vi "Controle_Manip_Main_GUI_Backup1.vi"() -> ()   [LabVIEW 2019]
doc: "VI for micro-photoluminescence setup in GH013 to study the emission properties of single nanoemitters in the visible range."
uses:
  subVIs/TypeDefs/AcqMode.ctl
  D:/Users/manip-thz/Documents/Controle_Manip_2020/Thorlabs.MotionControl.Controls.dll
  Thorlabs.MotionControl.Controls.dll
  D:/Users/manip-thz/Documents/Controle_Manip_2020/Thorlabs.MotionControl.KCube.SolenoidCLI.dll
  Thorlabs.MotionControl.KCube.SolenoidCLI.dll
  D:/Users/manip-thz/Documents/Controle_Manip_2020/Thorlabs.MotionControl.KCube.PiezoCLI.dll
  Thorlabs.MotionControl.KCube.PiezoCLI.dll
  subVIs/Light Field/lightfield-automation-labview/LightField Automation.lvclass
  subVIs/Light Field/lightfield-automation-labview/VIs/TypeDefs/OpticalPortLocation.ctl
  System.Windows.Forms
  C:/Program Files/Thorlabs/Scientific Imaging/DCx Camera Support/Develop/DotNet/uc480DotNet.dll
  <vilib>/DAQmx/write.llb/DAQmx Write (Analog DBL 1Chan 1Samp).vi
  <vilib>/DAQmx/create/channels.llb/DAQmx Create Channel (AO-Voltage-Basic).vi
  <vilib>/DAQmx/miscellaneous.llb/DAQmx Fill In Error Info.vi
  subVIs/Newport/Newport ESP301/Newport ESP301.lvlib
panel:
  out "Thorcam Error":errorcluster caption="Error Out"
  out "ThorCam Reference":refnum<k24>
  out "Shutter Ctrls":u16(ring)
  out "Serial Number":string
  out "Scan XY Map Params":refnum<vi>[](array[refnum])
  in  "Diode Driver Error":errorcluster caption="error in (no error)" {"code" format="%.0x"}
  out "Color":u32(colorbox)=4980812
  out "Laser on?":bool
  out "Angles":dbl[](array[numeric])
  out "Scan Polar Params":refnum<vi>[](array[refnum])
  in  "ESP 301 Error":errorcluster
  in  "ESP300 Error":errorcluster
  out "Data":T1(array[cluster])
  out "Wavelength calibration":dbl[](array[numeric])
  out "LightField Automation error out":errorcluster
  out "LightField Automation out":refnum<class "LightField Automation.lvclass">
  out "Photodiode error out":errorcluster caption="error out" {"code" format="%.0x"}
  out "Photodiode handle out":refnum<visa-resource-name> caption="instrument handle out"
  out "KCubePiezoControl X Reference":refnum<k24>
  out "KCubePiezoDevice X Reference":refnum<k24>
  out "KCubePiezoDevice Y Reference":refnum<k24>
  out "KCubePiezoControl Y Reference":refnum<k24>
  out "KCubePiezoControl Z Reference":refnum<k24>
  out "KCubePiezoDevice Z Reference":refnum<k24>
  out "KCube Shutter Device Reference":refnum<k24>
  in  "Shutter mode":bool
  out "KCubeSolenoidControl Reference":refnum<k24>
  in  "Cryostat":enum16{"Montana", "Oxford"}(ring) caption="Cryo :"
  out "Excitation Power (uW)":dbl=0.2 caption="P    =" format="%#_3p"
  in  "Acq Time (ms)":dbl=500.0 caption="Acq Time :" min=0.0 max=360000.0 step=50.0
  in  "Auto< ?":bool
  in  "Acq Mode":T2=enum."Spectrum" caption="Acquire :"
  in  "Comment":string
  out "Log file":string caption="Status"
  in  "Experiment Name":string="B1802CF_QD0"
  in  "Experiment Graph Controls":T3(tab)
  in  "CCD 1D Spectrum Main  Cursor2WL 2 Mono 2":bool caption="CCD 1D Spectrum Main  Cursor2WL"
  in  "CCD 1D Spectrum Main  Cursor2WL 1 Mono 2":bool caption="CCD 1D Spectrum Main  Cursor2WL"
  in  "CCD 1D Spectrum Main  Cursor2WL 2 Mono 1":bool caption="CCD 1D Spectrum Main  Cursor2WL"
  in  "CCD 1D Spectrum Main  Cursor2WL 1 Mono 1":bool caption="CCD 1D Spectrum Main  Cursor2WL"
  out "CCD 1D Spectrum Main Cursor 1 nm":dbl caption="nm"
  out "CCD 1D Spectrum Main Cursor 2 nm":dbl caption="nm"
  in  "Full scale":bool
  in  "Acquire Continuous Spectrum":bool
  in  "Acquire Spectrum":bool
  out "CCD 2D Image Main":dbl[][](graph)
  in  "Save Spectrum N":bool
  in  "Save Spectrum":bool
  out "CCD 1D Spectrum Main":cluster{dbl[], dbl[]}(graph)
  in  "Stop continuous":bool
  out "CCD 1D Spectrum Main Energy Scale":cluster{dbl[], dbl[]}(graph)
  out "CCD 1D Spectrum Main Cursor":dbl caption="eV" format="%#_6p"
  out "CCD 1D Spectrum Main Cursor 2":dbl caption="eV" format="%#_6p"
  out "CCD 1D Spectrum Main deltaE":dbl caption="eV" format="%#_3p"
  out "CCD 1D Spectrum Main deltanm":dbl caption="m" format="%#_3p"
  out "XY Intensity Map":dbl[][](graph)=[[3.904687043201515e-13, 6.684989195773002e-11, 3.649880430807626e-09, 6.355065252727497e-08, 3.5287820878809013e-07, 6.248749509463085e-07, 3.5287820878809013e-07, 6.355065252727497e-08, 3.649880430807626e-09, 6.684989195773002e-11, 3.904687043201515e-13], [6.684989195773002e-11, 1.1444983952148092e-08, 6.248749509463097e-07, 1.0880140221963334e-05, 6.041424029819161e-05, 0.0001069812317752422, 6.041424029819161e-05, 1.0880140221963334e-05, 6.248749509463097e-07, 1.1444983952148092e-08, 6.684989195773002e-11], [3.649880430807626e-09, 6.248749509463097e-07, 3.41170163237202e-05, 0.0005940355282204004, 0.003298505755939091, 0.005840977343195246, 0.003298505755939091, 0.0005940355282204004, 3.41170163237202e-05, 6.248749509463097e-07, 3.649880430807626e-09], [6.355065252727497e-08, 1.0880140221963334e-05, 0.0005940355282204004, 0.01034317319661825, 0.05743261926761737, 0.10170139230422684, 0.05743261926761737, 0.01034317319661825, 0.0005940355282204004, 1.0880140221963334e-05, 6.355065252727497e-08], [3.5287820878809013e-07, 6.041424029819161e-05, 0.003298505755939091, 0.05743261926761737, 0.31890655732397044, 0.5647181220077593, 0.31890655732397044, 0.05743261926761737, 0.003298505755939091, 6.041424029819161e-05, 3.5287820878809013e-07], [6.248749509463085e-07, 0.0001069812317752422, 0.005840977343195246, 0.10170139230422684, 0.5647181220077593, 1.0, 0.5647181220077593, 0.10170139230422684, 0.005840977343195246, 0.0001069812317752422, 6.248749509463085e-07], [3.5287820878809013e-07, 6.041424029819161e-05, 0.003298505755939091, 0.05743261926761737, 0.31890655732397044, 0.5647181220077593, 0.31890655732397044, 0.05743261926761737, 0.003298505755939091, 6.041424029819161e-05, 3.5287820878809013e-07], [6.355065252727497e-08, 1.0880140221963334e-05, 0.0005940355282204004, 0.01034317319661825, 0.05743261926761737, 0.10170139230422684, 0.05743261926761737, 0.01034317319661825, 0.0005940355282204004, 1.0880140221963334e-05, 6.355065252727497e-08], [3.649880430807626e-09, 6.248749509463097e-07, 3.41170163237202e-05, 0.0005940355282204004, 0.003298505755939091, 0.005840977343195246, 0.003298505755939091, 0.0005940355282204004, 3.41170163237202e-05, 6.248749509463097e-07, 3.649880430807626e-09], [6.684989195773002e-11, 1.1444983952148092e-08, 6.248749509463097e-07, 1.0880140221963334e-05, 6.041424029819161e-05, 0.0001069812317752422, 6.041424029819161e-05, 1.0880140221963334e-05, 6.248749509463097e-07, 1.1444983952148092e-08, 6.684989195773002e-11], [3.904687043201515e-13, 6.684989195773002e-11, 3.649880430807626e-09, 6.355065252727497e-08, 3.5287820878809013e-07, 6.248749509463085e-07, 3.5287820878809013e-07, 6.355065252727497e-08, 3.649880430807626e-09, 6.684989195773002e-11, 3.904687043201515e-13]]
  out "CCD 2D Image XY Map":dbl[][](graph)
  out "CCD 1D Spectrum XY Map":dbl[][](graph)
  out "Polarisation 2D Image":dbl[][](graph)
  out "Polarisation 1D Spectrum":cluster{dbl[], dbl[]}(graph) caption="360.0°"
  out "Polarisation 1D Spectrum Energy Scale":cluster{dbl[], dbl[]}(graph)
  in  "ThorCam Init":bool
  in  "ThorCam Visu":refnum<k24>(container)
  in  "Conv/Energy (eV)":dbl caption="Energy :" format="%#_6p"
  in  "Conv/Wavelength (nm)":dbl caption="Wavelength :"
  in  "Conv/Wavenumber (m-1)":dbl caption="Wavenumber :"
  in  "Conv/Time (s)":dbl caption="Time :" format="%#_6p"
  in  "Laser Diode Current Set":dbl(slide)=0.02 caption="Laser Power (a.u.)" min=0.02 max=0.061 scale=0.02..0.05 scale format="%#_3g"
  in  "Laser on? Control":bool
  in  "Diode Driver COM":refnum<visa-resource-name>="USB0::0x1313::0x804F::M00549740::INSTR"
  in  "Laser Comm On?":bool
  in  "KCube Shutter On?":bool
  in  "KCubes Piezo On?":bool
  in  "LightField On?":bool
  in  "PM16-120 On?":bool
  in  "ESP 300 On?":bool
  in  "ESP 301 On?":bool
  in  "FSM 300 On?":bool
  in  "ESP 300 COM Port":refnum<visa-resource-name>="COM1" caption="COM Port"
  in  "Excitation Wavelength (nm)":dbl=400.0 caption="Exc WL (nm)" min=400.0 max=1100.0 step=1.0
  out "Photodiode Status":bool caption="Status"
  in  "Photodiode COM Port":refnum<visa-resource-name>="USB0::0x1313::0x807B::190927109::INSTR" caption="COM Port"
  in  "ESP 301 COM Port":refnum<visa-resource-name>="COM4" caption="COM Port"
  in  "FSM Y Axis":tag="cDAQ2Mod1/ao1"
  in  "FSM X Axis":tag="cDAQ2Mod1/ao2"
  in  "Slit Width (mm)":dbl
  out "Initialise all devices?":bool caption="OK"
  in  "TEC Output":bool
  out "TEC Temperature":dbl caption="TEC Temp" format="%#_4f"
  out "Laser Safety":u16(ring)
  in  "Stop Everything & Quit?":bool
  in  "Excitation Source":enum16{"P", "CW"}(ring)=enum."CW" caption="Laser"
  in  "Temperature (K)":dbl=5.0 caption="T ="
  in  "Experimental parameters tab":T4(tab)
  in  "Center Wavelength (nm) Mono 2":dbl
  in  "Mono2 Motor Position":dbl
  out "Mono2 On":bool
  in  "CCD ROI":T5(ring)
  in  "Spectrum Step Wavelength (nm)":dbl=490.12 caption="Step WL (nm)"
  in  "Spectrum End Wavelength (nm)":dbl=490.12 caption="End WL (nm)"
  in  "Spectrum Start Wavelength (nm)":dbl=490.12 caption="Start WL (nm)"
  in  "Accumulations":dbl=1.0 caption="Accum."
  in  "Background substract":enum16{"None", "Shutter"}(ring) caption="Bkg substract"
  in  "Exit mirror":enum16{"CCD", "APD"}(ring)
  in  "Center Wavelength (nm)":dbl=490.12 caption="Center WL (nm)"
  in  "Exposure Time (ms)":dbl=500.0 caption="Exp Time (ms)" min=0.0 max=360000.0 step=50.0
  in  "Grating":string(combo)="[h-vis,2400][0][0]"
  out "CCD T°  (°C)":dbl
  in  "LF Visible":bool=TRUE
  out "Exit Port Location":T6 items=["None"=1, "SideEntrance"=2, "FrontEntrance"=3, "SideExit"=5, "FrontExit"=4]
  out "Scan Spectrum Progess Bar":u8(slide) scale=0.0..100.0
  in  "Stop XY Map":bool
  out "Scan X Readout (V)":dbl caption="X Readout (V)" min=-10.0 max=10.0
  out "Scan Y Readout (V)":dbl caption="Y Readout (V)" min=-10.0 max=10.0
  out "Scan XY Map Progess Bar":u8(slide) scale=0.0..100.0
  in  "Scan Y Tot. Length":dbl caption="Y Length"
  in  "Scan X Tot. Length (V)":dbl caption="X Length (V)"
  in  "Scan Y Num. Pts":dbl caption="Y # Pts"
  in  "Scan X Num. Pts":dbl caption="X # Pts"
  in  "Scan Y Res. (V)":dbl caption="Res. Y (V)"
  in  "Scan X Res. (V)":dbl caption="Res. X (V)"
  in  "Scan Y Center (V)":dbl caption="Y Center (V)"
  in  "Scan X Center (V)":dbl caption="X Center (V)"
  in  "FSM Home":bool
  in  "FSM Right":bool
  in  "FSM Left":bool
  in  "FSM Down":bool
  in  "FSM Up":bool
  in  "FSM X Axis Pos":dbl min=-10.0 max=10.0
  in  "FSM Y Axis Pos":dbl min=-10.0 max=10.0
  in  "FSM Axis Step":dbl=0.1
  in  "Save XY Map":bool
  in  "Acquire XY Map":bool
  in  "Scanning Mode":T7(ring) caption="Mode"
  in  "Scan Fast Axis":enum16{"Y", "X"}(ring)=enum."X" caption="Fast Axis"
  out "RotStage Det Angle Readout (°)":dbl=2.0 caption="Readout (°)" min=-360.0 max=360.0 format="%#_4g"
  out "RotStage Exc Angle Readout (°)":dbl=2.0 caption="Readout (°)" min=-360.0 max=360.0 format="%#_4g"
  in  "Acquire Polarisation":bool
  in  "RotStage Det Angle Step (°)":dbl=10.0 caption="Step (°)"
  in  "RotStage Exc Angle Step (°)":dbl=10.0 caption="Step (°)"
  in  "RotStage Det Jog Forward":bool
  in  "RotStage Exc Jog Forward":bool
  in  "RotStage Det Jog Backward":bool
  in  "RotStage Det Home":bool caption="Home"
  in  "RotStage Exc Home":bool caption="Home"
  in  "RotStage Det Angle (°)":dbl=2.0 caption="Target (°)" min=-360.0 max=360.0 format="%#_4g"
  in  "RotStage Exc Angle (°)":dbl=2.0 caption="Target (°)" min=-360.0 max=360.0 format="%#_4g"
  in  "RotStage Exc Jog Backward":bool
  in  "Polar Start Angle (°)":dbl caption="Start angle (°)" min=0.0 max=360.0 step=10.0
  in  "Polar End Angle (°)":dbl=360.0 caption="End Angle (°)" min=0.0 max=360.0 step=10.0
  in  "Polar Step Angle (°)":dbl=10.0 caption="Step Angle (°)" min=1.0 max=360.0
  in  "Polar mode":u16(ring)=3 caption="Rotate polarisation" items=["Excitation"=3, "Detection"=2]
  in  "Save Polarisation":bool
  out "Scan Polarisation Progess Bar":u8(slide) scale=0.0..100.0
  in  "RotStage Det Velocity (°/s)":dbl=2.0 caption="Velocity (°/s)" min=1.0 max=20.0 step=1.0
  in  "RotStage Exc Velocity (°/s)":dbl=2.0 caption="Velocity (°/s)" min=1.0 max=20.0 step=1.0
  out "Newport Linear Translation Stage Position Readout (mm)":dbl caption="Readout (mm)" min=-8.0 max=392.0
  in  "Newport Linear Translation Stage Step (mm)":dbl=5.0 caption="Step (mm)"
  in  "Delay Line Position (mm)":dbl caption="Delay line position (mm)"
  in  "Newport Linear Translation Stage Position (mm)":dbl caption="Target (mm)" min=-8.0 max=392.0
  out "Scan Linear Stage Progess Bar":u8(slide) scale=0.0..100.0
  in  "Newport Linear Translation Stage Home":bool caption="Home"
  in  "Newport Linear Translation Stage Jog Forward":bool
  in  "Newport Linear Translation Stage Jog Backward":bool
  in  "Newport Linear Translation Stage Velocity (mm/s)":dbl=1.0 caption="Velocity (mm/s)" min=1.0 max=100.0 step=1.0
  in  "KCubePiezoControl Z":refnum<k24>(container) caption="Focus"
  in  "KCubePiezoControl X":refnum<k24>(container) caption="Lateral"
  in  "KCubePiezoControl Y":refnum<k24>(container) caption="Vertical"
  in  "KCubeSolenoidControl":refnum<k24>(container)
  in  "Shutter Mode":i32(ring)=1 items=["Manual"=1, "SingleToggle"=2, "AutoToggle"=3, "Triggered"=4]
  # "ms"
  # "K"
  # "laser"
  # "exc"
  # "W"
  # "Mono 1"
  # "Mono 2"
  # "--|--"
  # "CenterWL"
  # "l   ="
  # "E  ="
  # "DE ="
  # "1"
  # "1"
  # "--|--"
  # "Dl ="
  # "CenterWL"
  # "l   ="
  # "E   ="
  # "2"
  # "2"
  # "Absolute conversions"
  # "change one value manually and the others will update automatically"
  # "Relative conversions"
  # "eV"
  # "nm"
  # "-1"
  # "cm"
  # "s"
  # "Thorlabs Laser Diode Driver CLD1010"
  # "Newport FSM-300-01"
  # "Newport ESP 301"
  # "Newport ESP 300"
  # "Thorlabs PM16-120"
  # "Thorlabs Shutter SH05"
  # "Thorlabs NanoMax + 3 Axis Piezos"
  # "Princeton HRS-500 + Pixis"
  # "min"
  # "max"
  # "Controls"
  # "Scans"
  # "add functionnality spectrum with APD 1 or APD 2\nwith option AcqMode (with frw&bckw talk to Exit mirror)"
  # "Possibly add a slit size option to determine the resolution"
  # "Controls"
  # "Scans"
  # "Controls"
  # "Scans"
  # "Excitation"
  # "Detection"
  # "Controls"
  # "Scans"
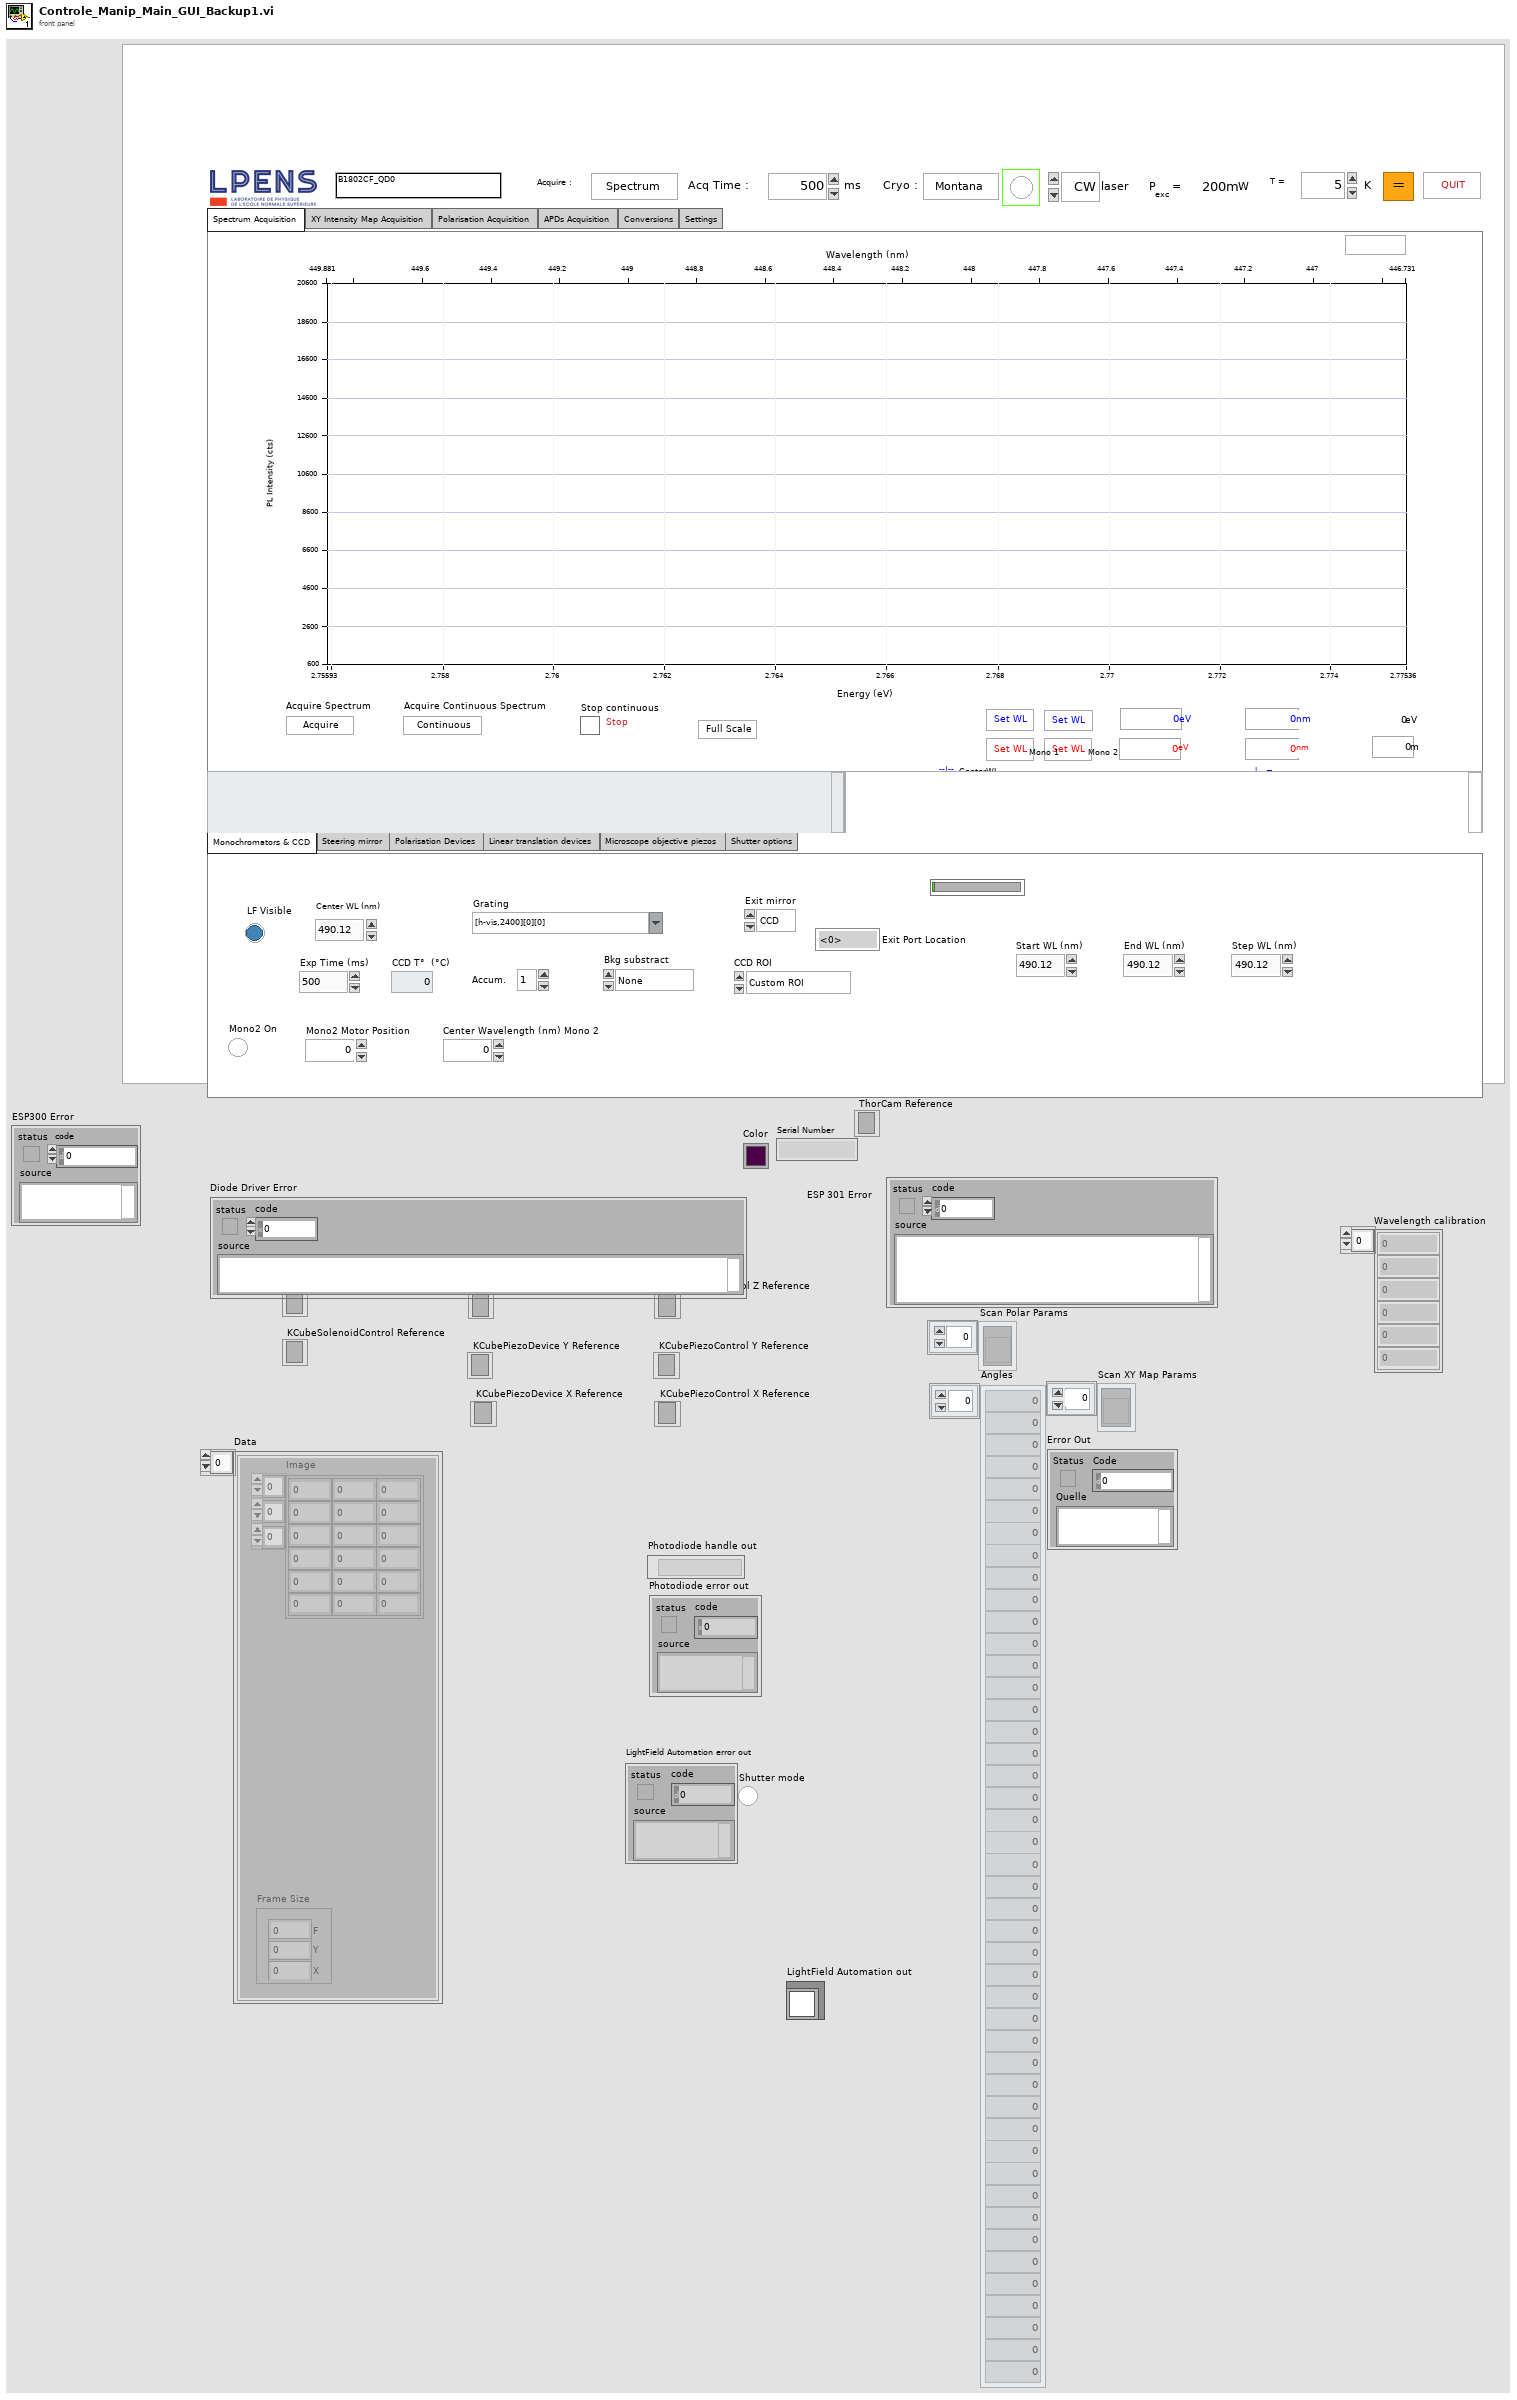
[diagram p1: front panel]
types:
  T1 = cluster{"Image":dbl[][][], "Frame Size":cluster{"F":i32, "Y":i32, "X":i32}}[]
  T2 = typedef "AcqMode.ctl" = enum16{"Image", "Spectrum", "APD 1", "APD 2", "APD 1+2"}
  T3 = enum32{"Spectrum Acquisition", "XY Intensity Map Acquisition", "Polarisation Acquisition", "APDs Acquisition", "Conversions", "Settings"}
  T4 = enum32{"Monochromators & CCD", "Steering mirror", "Polarisation Devices", "Linear translation devices", "Microscope objective piezos", "Shutter options"}
  T5 = enum16{"Custom ROI", "Full sensor", "Binned full sensor"}
  T6 = typedef "LightField Automation.lvclass/OpticalPortLocation.ctl" = i32
  T7 = enum16{"Default", "Snail", "Random", "Snake", "Line"}
  T8 = enum16{"Spectre", "Polarisation", "XY Intensity Map"}
  T9 = enum16{"XY Intensity Map", "Polarisation", "Spectrum"}
  T10 = typedef "LVRangeTypeDef.ctl" = cluster{"Minimum":dbl, "Maximum":dbl, "Increment":dbl, "Minor Increment":dbl, "Start":dbl}
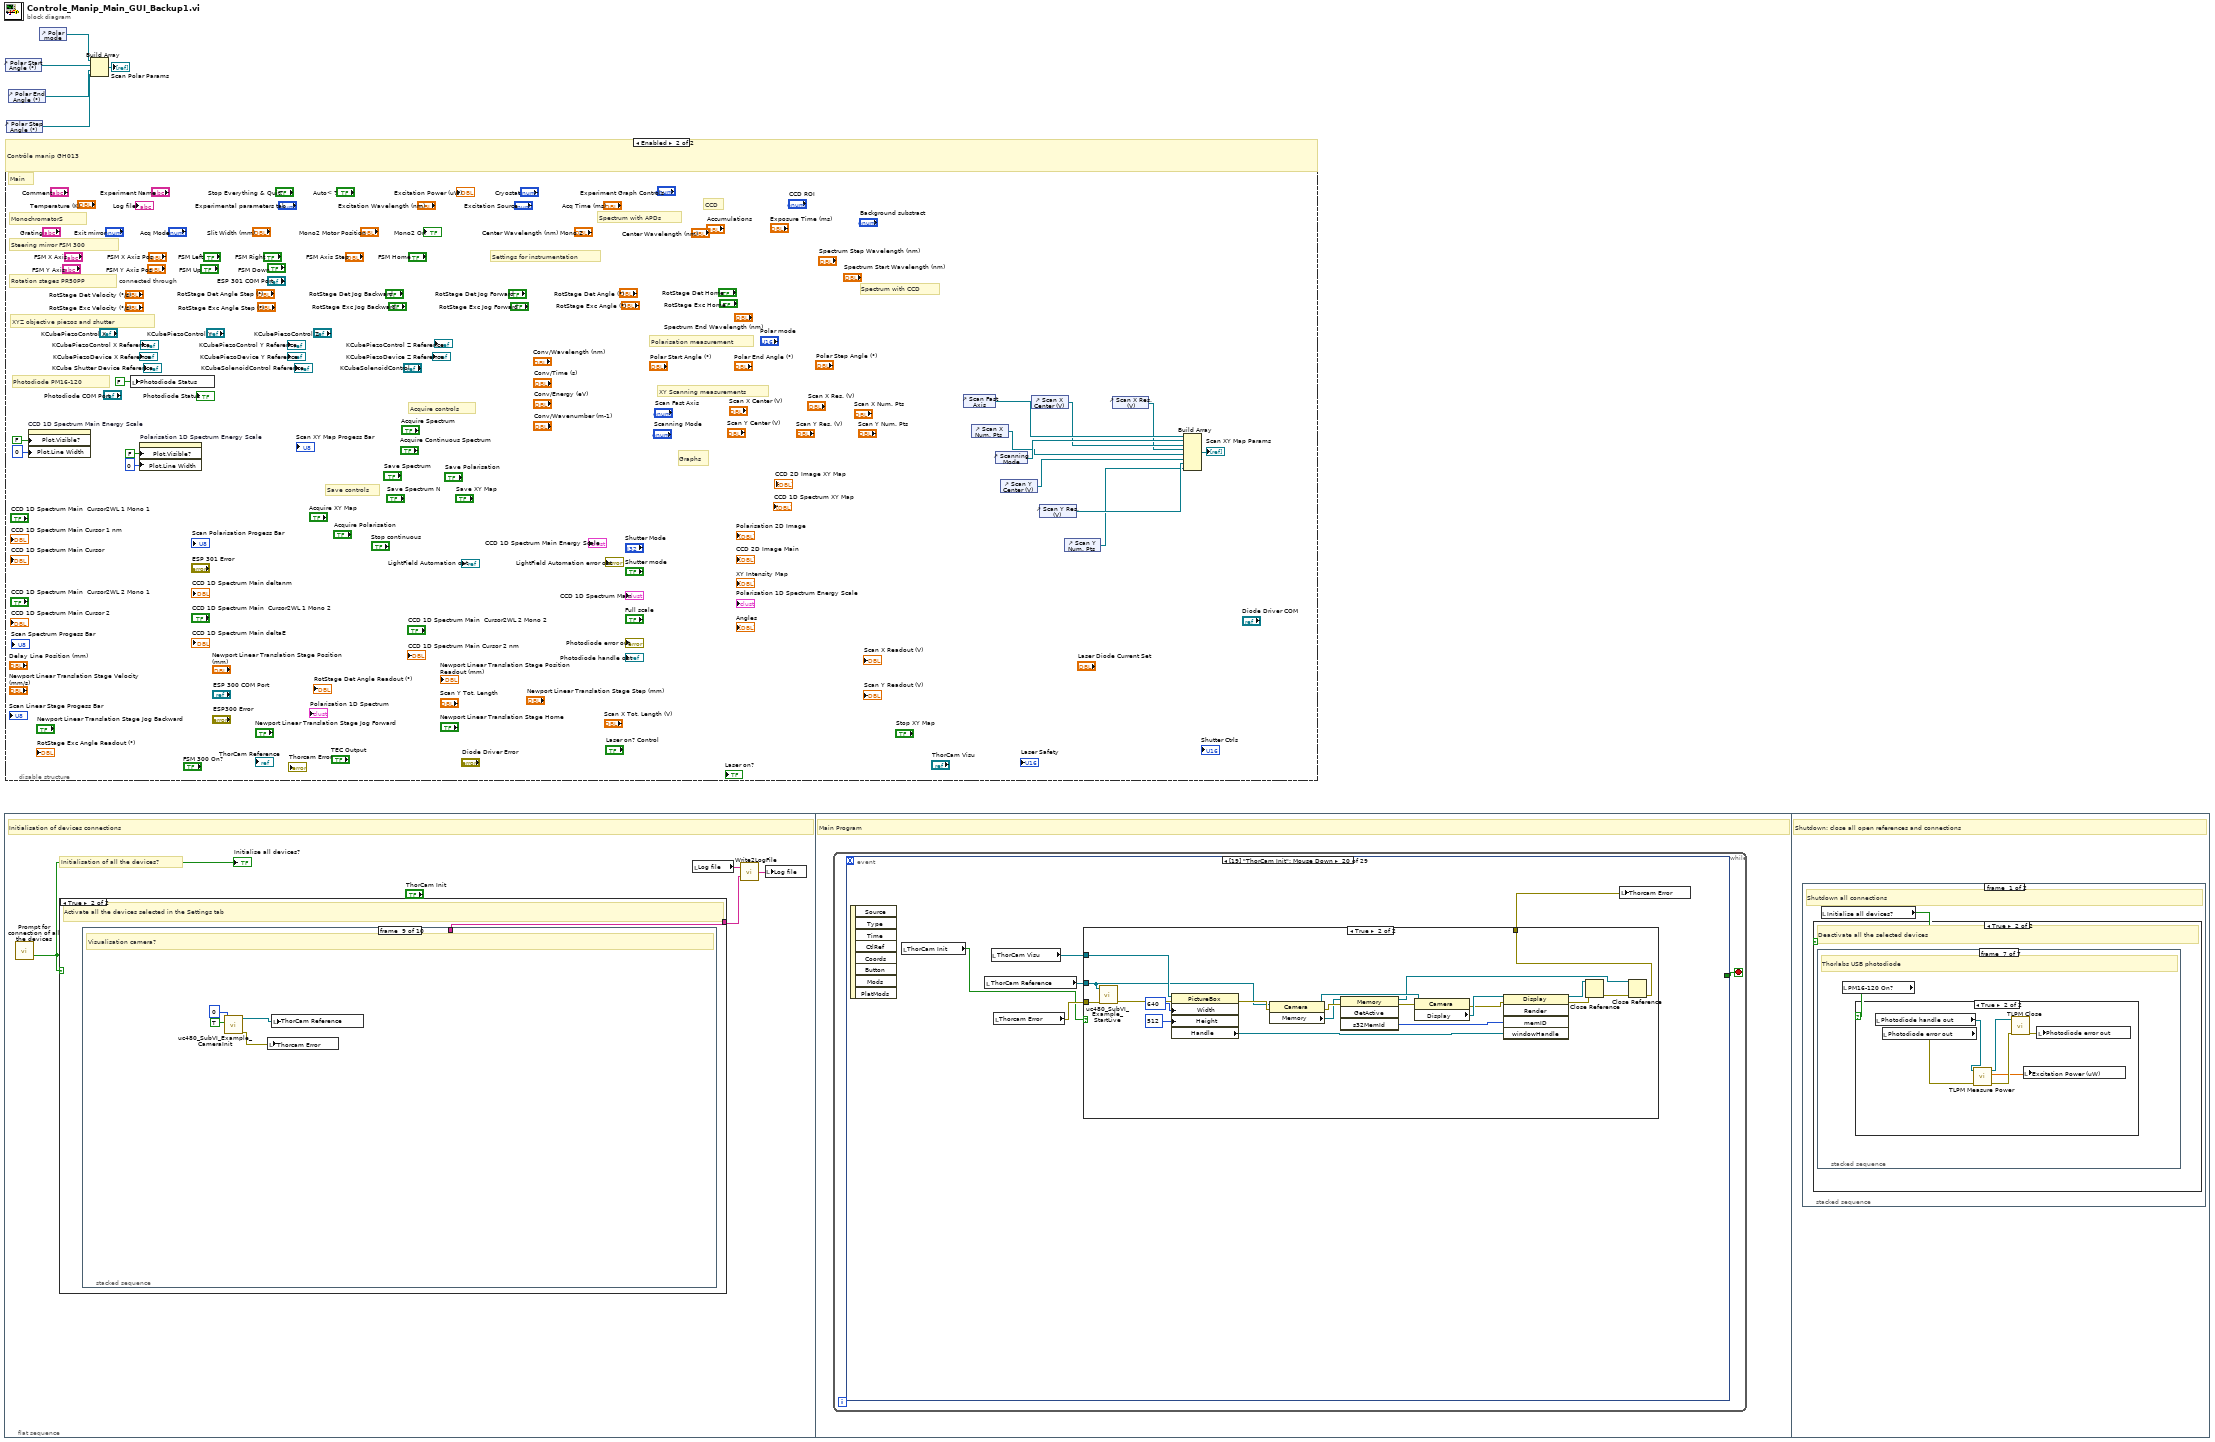
[diagram p0: block diagram]
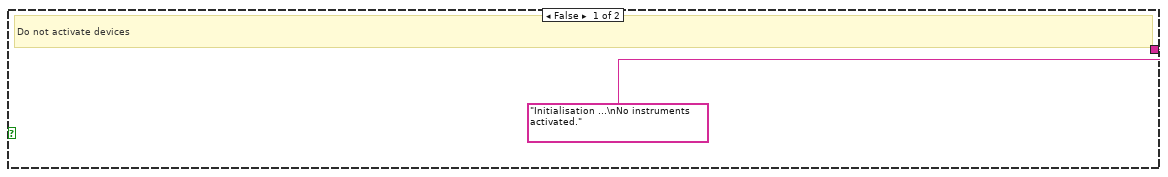
[diagram p3: hidden frame]
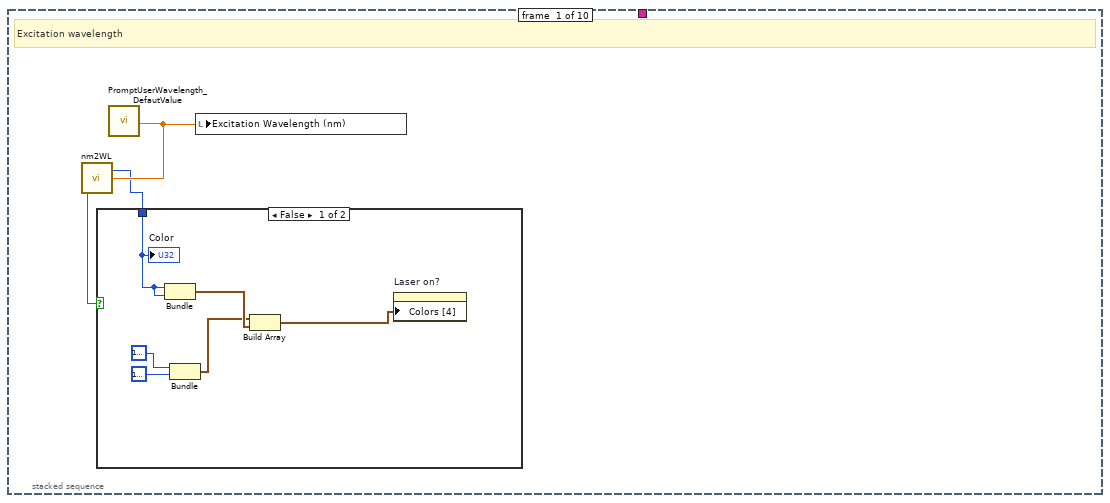
[diagram p4: hidden frame]
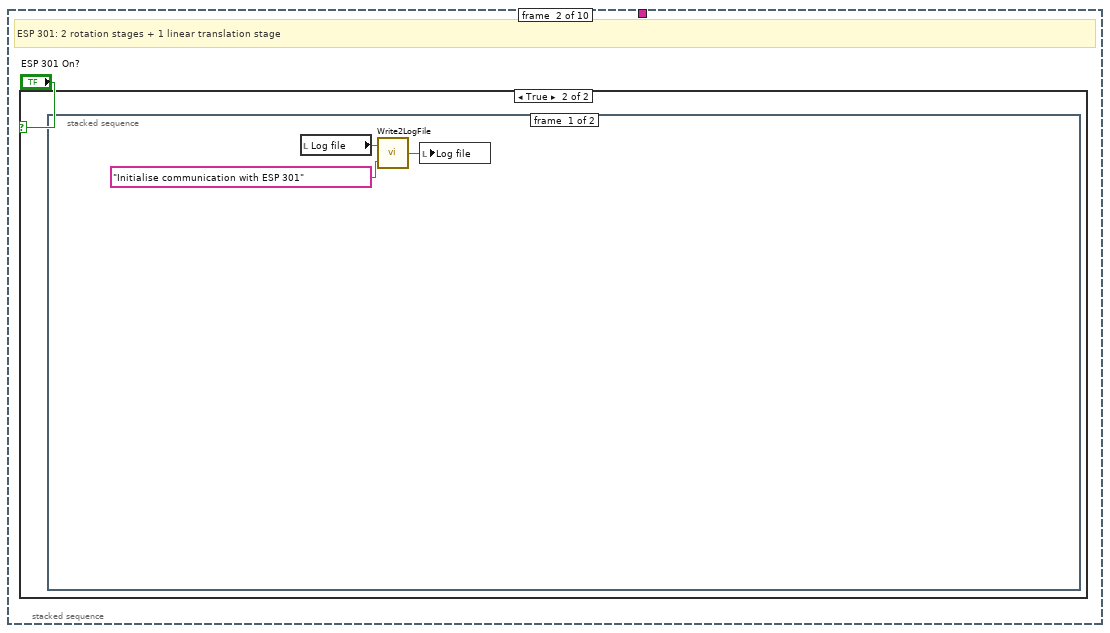
[diagram p6: hidden frame]
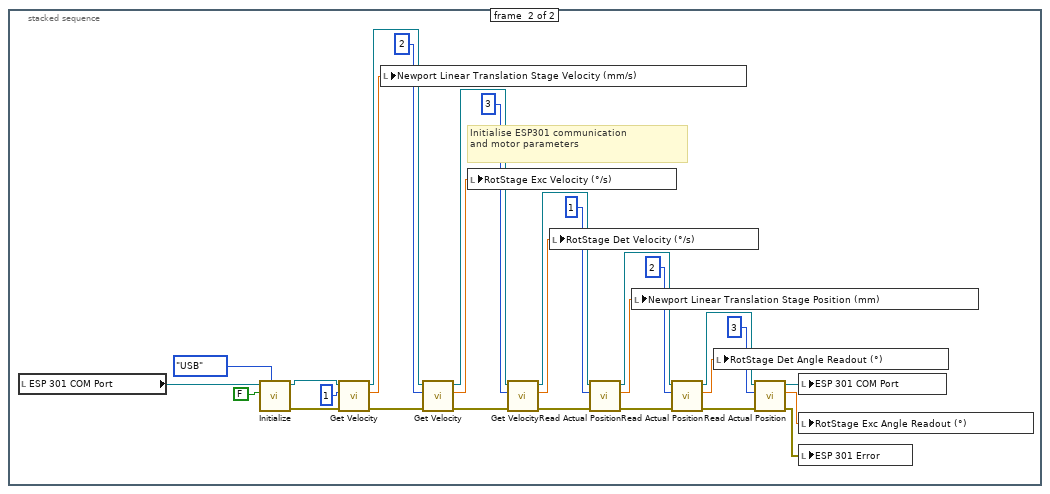
[diagram p8: hidden frame]
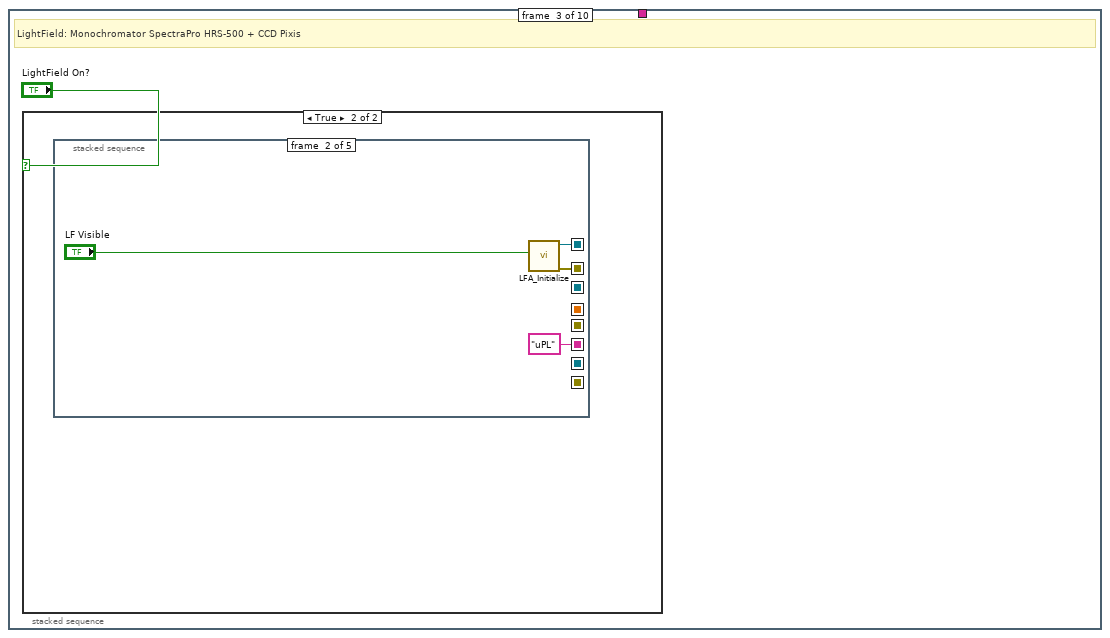
[diagram p9: hidden frame]
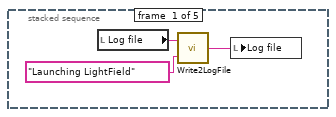
[diagram p11: hidden frame]
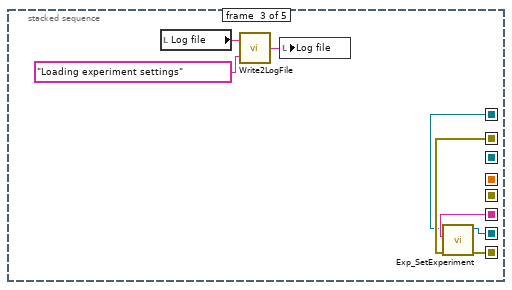
[diagram p12: hidden frame]
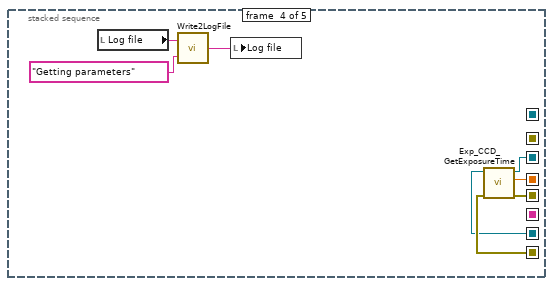
[diagram p13: hidden frame]
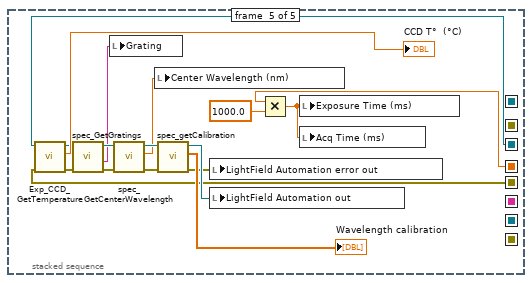
[diagram p14: hidden frame]
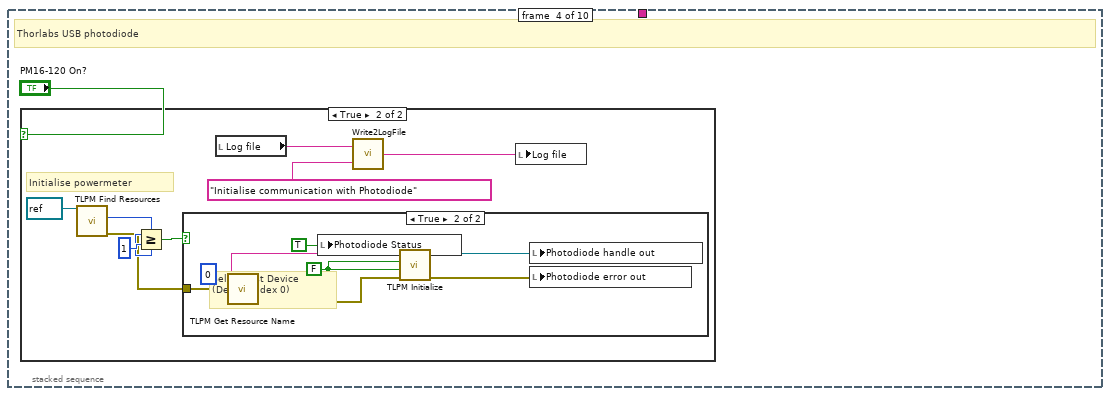
[diagram p15: hidden frame]
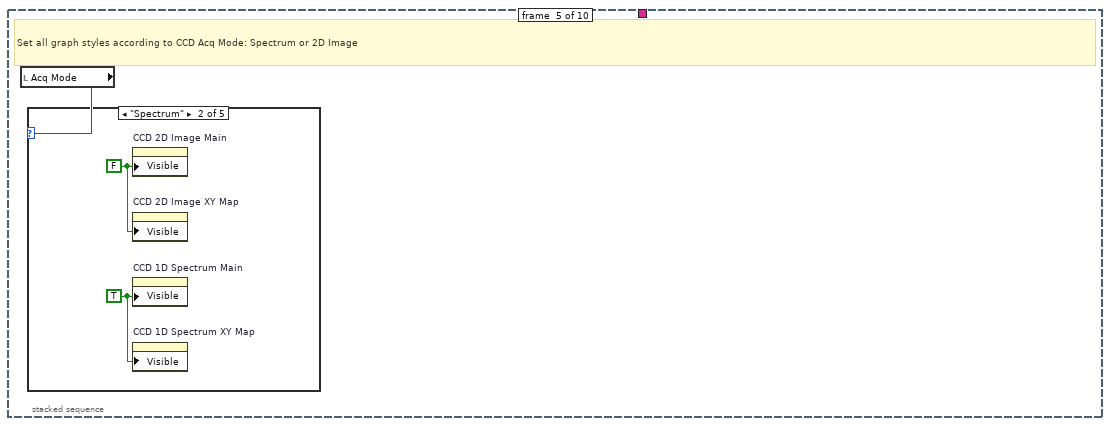
[diagram p18: hidden frame]
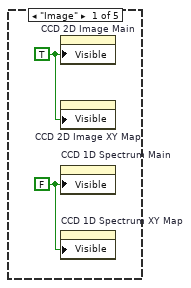
[diagram p19: hidden frame]
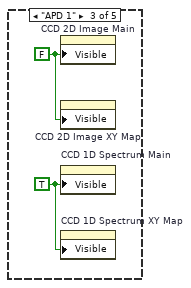
[diagram p20: hidden frame]
diagram:
  n1 = flat-sequence {
    frame #0 {
      # "Initialisation of all the devices?"
      # "Initialisation of devices connections"
      n2 = call "Prompt for connection of all the devices"() -> ("OK"=w6:bool)  [unwired: 18 in, 1 out]
      "Initialise all devices?" <- w6
      n3 = case shown="True" w6 {
        tunnel: ["Initialisation ...\nNo instruments activated." w11] -> w8
        frame False {
          # "Do not activate devices"
        }
        frame True {
          # "Activate all the devices selected in the Settings tab"
          n4 = stacked-sequence {
            tunnel: [_ _ _ _ _ _ _ _ _ "All devices activated !"] -> w11
            frame #0 {
              # "Excitation wavelength"
              n5 = call "PromptUserWavelength_DefautValue.vi"() -> ("Wavelength"=w14:dbl)  [unwired: 17 in, 2 out]
              n6 = call "nm2WL.vi"("Wavelength (380 - 780)"=w14) -> ("Color"=w12:u32, "Out Of Range"=w13:bool)
              n7 = case shown="False" w13 {
                tunnel: w12 -> [w18 _]
                frame False {
                  n8 = Bundle("Color"=w18, "Color"=w18) -> (w17:cluster{"Color":u32, "Color":u32})  [unwired: 1 in]
                  n9 = Bundle(u32 16777216, u32 16777216) -> (w16:cluster{u32, u32})  [unwired: 1 in]
                  n10 = Build Array(w16, w17) -> (w15:cluster{"Color":u32, "Color":u32}[])
                  n11 = property on="Laser on?" class="Bool (strict)"("Colors [4]"=w15) -> ()  [unwired: 2 in, 2 out]
                  "Color" <- w18
                }
                frame True {
                }
              }
              n12 = local write "Excitation Wavelength (nm)"(w14) -> ()
            }
            frame #1 {
              # "ESP 301: 2 rotation stages + 1 linear translation stage"
              n13 = case shown="True" "ESP 301 On?" {
                frame False {
                }
                frame True {
                  n14 = stacked-sequence {
                    frame #0 {
                      n15 = local read "Log file"() -> (w24:string)
                      n16 = call "Write2LogFile.vi"("Add to log file"="Initialise communication with ESP 301", "Log file before"=w24) -> ("Log file after"=w22:string)
                      n17 = local write "Log file"(w22) -> ()
                    }
                    frame #1 {
                      # "Initialise ESP301 communication\nand motor parameters"
                      n18 = local read "ESP 301 COM Port"() -> (w33:refnum<visa-resource-name>)
                      n19 = call "Initialize.vi"("VISA resource name"=w33, "ID Query (True)"=FALSE, "Serial Link (RS232)"=enum16{"RS232", "USB"}."USB") -> ("VISA resource name out"=w39:refnum<visa-resource-name>, "error out"=w38:errorcluster)  [unwired: 6 in]
                      n20 = call "Get Velocity.vi"("error in (no error)"=w38, "Axis (1)"=1, "VISA resource name"=w39) -> ("error out"=w36:errorcluster, "Velocity (units/s)"=w40:dbl, "VISA resource name out"=w35:refnum<visa-resource-name>)  [unwired: 2 in]
                      n21 = local write "Newport Linear Translation Stage Velocity (mm/s)"(w40) -> ()
                      n22 = call "Get Velocity.vi"("error in (no error)"=w36, "Axis (1)"=2, "VISA resource name"=w35) -> ("error out"=w37:errorcluster, "Velocity (units/s)"=w42:dbl, "VISA resource name out"=w34:refnum<visa-resource-name>)  [unwired: 2 in]
                      n23 = local write "RotStage Exc Velocity (°/s)"(w42) -> ()
                      n24 = call "Get Velocity.vi"("error in (no error)"=w37, "Axis (1)"=3, "VISA resource name"=w34) -> ("error out"=w44:errorcluster, "Velocity (units/s)"=w41:dbl, "VISA resource name out"=w43:refnum<visa-resource-name>)  [unwired: 2 in]
                      n25 = local write "RotStage Det Velocity (°/s)"(w41) -> ()
                      n26 = call "Read Actual Position.vi"("error in (no error)"=w44, "Axis (1)"=1, "VISA resource name"=w43) -> ("error out"=w50:errorcluster, "Position (units)"=w51:dbl, "VISA resource name out"=w49:refnum<visa-resource-name>)  [unwired: 2 in]
                      n27 = local write "Newport Linear Translation Stage Position (mm)"(w51) -> ()
                      n28 = call "Read Actual Position.vi"("error in (no error)"=w50, "Axis (1)"=2, "VISA resource name"=w49) -> ("error out"=w47:errorcluster, "Position (units)"=w45:dbl, "VISA resource name out"=w48:refnum<visa-resource-name>)  [unwired: 2 in]
                      n29 = local write "RotStage Det Angle Readout (°)"(w45) -> ()
                      n30 = call "Read Actual Position.vi"("error in (no error)"=w47, "Axis (1)"=3, "VISA resource name"=w48) -> ("error out"=w53:errorcluster, "Position (units)"=w46:dbl, "VISA resource name out"=w52:refnum<visa-resource-name>)  [unwired: 2 in]
                      n31 = local write "ESP 301 COM Port"(w52) -> ()
                      n32 = local write "RotStage Exc Angle Readout (°)"(w46) -> ()
                      n33 = local write "ESP 301 Error"(w53) -> ()
                    }
                  }
                }
              }
            }
            frame #2 {
              # "LightField: Monochromator SpectraPro HRS-500 + CCD Pixis"
              n34 = case shown="True" "LightField On?" {
                frame False {
                }
                frame True {
                  n35 = stacked-sequence {
                    seq-local: [_ "uPL" ("ExperimentName") _ _ _] -> [_ _ w68 _ _]
                    seq-local: [_ w60 _ _ _] -> [_ _ w69 _ _]
                    seq-local: [_ w59 _ _ _] -> [_ _ w67 _ _]
                    seq-local: [_ _ w66 _ _] -> [_ _ _ w77 _]
                    seq-local: [_ _ w65 _ _] -> [_ _ _ w76 _]
                    seq-local: [_ _ _ w71 _] -> [_ _ _ _ w79]
                    seq-local: [_ _ _ w72 _] -> [_ _ _ _ w80]
                    seq-local: [_ _ _ w70 _] -> [_ _ _ _ w78]
                    frame #0 {
                      n36 = local read "Log file"() -> (w56:string)
                      n37 = call "Write2LogFile.vi"("Add to log file"="Launching LightField", "Log file before"=w56) -> ("Log file after"=w57:string)
                      n38 = local write "Log file"(w57) -> ()
                    }
                    frame #1 {
                      n39 = call "LFA_Initialize.vi"("Is Visible?"="LF Visible") -> ("error out"=w60:errorcluster, "LightField Automation out"=w59:refnum<class "LightField Automation.lvclass">)  [unwired: 9 in]
                    }
                    frame #2 {
                      n40 = local read "Log file"() -> (w62:string)
                      n41 = call "Write2LogFile.vi"("Add to log file"="Loading experiment settings", "Log file before"=w62) -> ("Log file after"=w63:string)
                      n42 = local write "Log file"(w63) -> ()
                      n43 = call "Exp_SetExperiment.vi"("error in (no error)"=w69, "ExperimentName"=w68, "LightField Automation in"=w67) -> ("error out"=w66:errorcluster, "LightField Automation out"=w65:refnum<class "LightField Automation.lvclass">)  [unwired: 7 in]
                    }
                    frame #3 {
                      n44 = local read "Log file"() -> (w75:string)
                      n45 = call "Write2LogFile.vi"("Add to log file"="Getting parameters", "Log file before"=w75) -> ("Log file after"=w74:string)
                      n46 = local write "Log file"(w74) -> ()
                      n47 = call "Exp_CCD_GetExposureTime.vi"("error in (no error)"=w77, "LightField Automation in"=w76) -> ("error out"=w71:errorcluster, "Exposure Time (s)"=w70:dbl, "LightField Automation out"=w72:refnum<class "LightField Automation.lvclass">)  [unwired: 7 in]
                    }
                    frame #4 {
                      n48 = call "Exp_CCD_GetTemperature.vi"("error in (no error)"=w79, "LightField Automation in"=w80) -> ("error out"=w84:errorcluster, "Temperature (°C)"=→"CCD T°  (°C)":dbl, "LightField Automation out"=w83:refnum<class "LightField Automation.lvclass">)  [unwired: 7 in]
                      n49 = call "spec_GetGratings.vi"("error in (no error)"=w84, "LightField Automation in"=w83) -> ("error out"=w93:errorcluster, "Current Grating"=w86:string, "LightField Automation out"=w94:refnum<class "LightField Automation.lvclass">)  [unwired: 6 in, 1 out]
                      n50 = local write "Grating"(w86) -> ()
                      n51 = call "spec_GetCenterWavelength.vi"("error in (no error)"=w93, "LightField Automation in"=w94) -> ("error out"=w91:errorcluster, "Center Wavelength"=w87:dbl, "LightField Automation out"=w89:refnum<class "LightField Automation.lvclass">)  [unwired: 7 in]
                      n52 = local write "Center Wavelength (nm)"(w87) -> ()
                      n53 = call "spec_getCalibration.vi"("error in (no error)"=w91, "LightField Automation in"=w89) -> ("error out"=w82:errorcluster, "ColumnCalibration"=→"Wavelength calibration":dbl[], "LightField Automation out"=w90:refnum<class "LightField Automation.lvclass">)  [unwired: 7 in]
                      n54 = local write "LightField Automation error out"(w82) -> ()
                      n55 = local write "LightField Automation out"(w90) -> ()
                      n56 = Multiply(x=w78, y=1000.0) -> (x*y=w88:dbl)
                      n57 = local write "Exposure Time (ms)"(w88) -> ()
                      n58 = local write "Acq Time (ms)"(w88) -> ()
                    }
                  }
                }
              }
            }
            frame #3 {
              # "Thorlabs USB photodiode"
              n59 = case shown="True" "PM16-120 On?" {
                frame False {
                }
                frame True {
                  # "Initialise powermeter"
                  n60 = call <instrlib>:"TLPM Find Resources.vi"("instrument handle"=refnum<visa-resource-name> refnum) -> ("error out"=w100:errorcluster, "Resource Count"=w102:u32)  [unwired: 8 in, 1 out]
                  n61 = Greater Or Equal?(x=w102, y=1) -> (x >= y?=w101:bool)
                  n62 = case shown="True" w101 {
                    tunnel: w100 -> [_ w111]
                    frame False {
                    }
                    frame True {
                      w110 = FALSE ("Reset Device (Reset Device)")
                      # "Select first Device\n(Device Index 0)"
                      n63 = call <instrlib>:"TLPM Get Resource Name.vi"("error in (no error)"=w111, "Index (0)"=u32 0) -> ("error out"=w108:errorcluster, "Resource Name"=w109:string)  [unwired: 7 in, 1 out]
                      n64 = local write "Photodiode Status"(TRUE) -> ()
                      n65 = call <instrlib>:"TLPM Initialize.vi"("error in (no error)"=w108, "Reset Device (Reset Device)"=w110, "ID Query (Do Query)"=w110, "resource name"=w109) -> ("error out"=w105:errorcluster, "instrument handle out"=w106:refnum<visa-resource-name>)  [unwired: 6 in]
                      n66 = local write "Photodiode handle out"(w106) -> ()
                      n67 = local write "Photodiode error out"(w105) -> ()
                    }
                  }
                  n68 = local read "Log file"() -> (w98:string)
                  n69 = call "Write2LogFile.vi"("Add to log file"="Initialise communication with Photodiode", "Log file before"=w98) -> ("Log file after"=w97:string)
                  n70 = local write "Log file"(w97) -> ()
                }
              }
            }
            frame #4 {
              # "Set all graph styles according to CCD Acq Mode: Spectrum or 2D Image"
              n71 = local read "Acq Mode"() -> (w112:T2)
              n72 = case shown="\"Spectrum\"" w112 {
                frame "Image" {
                  w114 = TRUE
                  w113 = FALSE
                  n73 = property on="CCD 2D Image Main" class="IntGraph (strict)"("Visible"=w114) -> ()  [unwired: 2 in, 2 out]
                  n74 = property on="CCD 2D Image XY Map" class="IntGraph (strict)"("Visible"=w114) -> ()  [unwired: 2 in, 2 out]
                  n75 = property on="CCD 1D Spectrum Main" class="XYGraph (strict)"("Visible"=w113) -> ()  [unwired: 2 in, 2 out]
                  n76 = property on="CCD 1D Spectrum XY Map" class="WFGraph (strict)"("Visible"=w113) -> ()  [unwired: 2 in, 2 out]
                }
                frame "Spectrum" {
                  w115 = FALSE
                  w116 = TRUE
                  n77 = property on="CCD 2D Image Main" class="IntGraph (strict)"("Visible"=w115) -> ()  [unwired: 2 in, 2 out]
                  n78 = property on="CCD 2D Image XY Map" class="IntGraph (strict)"("Visible"=w115) -> ()  [unwired: 2 in, 2 out]
                  n79 = property on="CCD 1D Spectrum Main" class="XYGraph (strict)"("Visible"=w116) -> ()  [unwired: 2 in, 2 out]
                  n80 = property on="CCD 1D Spectrum XY Map" class="WFGraph (strict)"("Visible"=w116) -> ()  [unwired: 2 in, 2 out]
                }
                frame "APD 1" {
                  w117 = FALSE
                  w118 = TRUE
                  n81 = property on="CCD 2D Image Main" class="IntGraph (strict)"("Visible"=w117) -> ()  [unwired: 2 in, 2 out]
                  n82 = property on="CCD 2D Image XY Map" class="IntGraph (strict)"("Visible"=w117) -> ()  [unwired: 2 in, 2 out]
                  n83 = property on="CCD 1D Spectrum Main" class="XYGraph (strict)"("Visible"=w118) -> ()  [unwired: 2 in, 2 out]
                  n84 = property on="CCD 1D Spectrum XY Map" class="WFGraph (strict)"("Visible"=w118) -> ()  [unwired: 2 in, 2 out]
                }
                frame "APD 2" {
                  w119 = FALSE
                  w120 = TRUE
                  n85 = property on="CCD 2D Image Main" class="IntGraph (strict)"("Visible"=w119) -> ()  [unwired: 2 in, 2 out]
                  n86 = property on="CCD 2D Image XY Map" class="IntGraph (strict)"("Visible"=w119) -> ()  [unwired: 2 in, 2 out]
                  n87 = property on="CCD 1D Spectrum Main" class="XYGraph (strict)"("Visible"=w120) -> ()  [unwired: 2 in, 2 out]
                  n88 = property on="CCD 1D Spectrum XY Map" class="WFGraph (strict)"("Visible"=w120) -> ()  [unwired: 2 in, 2 out]
                }
                frame "APD 1+2" {
                  w121 = FALSE
                  w122 = TRUE
                  n89 = property on="CCD 2D Image Main" class="IntGraph (strict)"("Visible"=w121) -> ()  [unwired: 2 in, 2 out]
                  n90 = property on="CCD 2D Image XY Map" class="IntGraph (strict)"("Visible"=w121) -> ()  [unwired: 2 in, 2 out]
                  n91 = property on="CCD 1D Spectrum Main" class="XYGraph (strict)"("Visible"=w122) -> ()  [unwired: 2 in, 2 out]
                  n92 = property on="CCD 1D Spectrum XY Map" class="WFGraph (strict)"("Visible"=w122) -> ()  [unwired: 2 in, 2 out]
                }
              }
            }
            frame #5 {
              # "KCubes: 1 Shutter + 3 Piezos for XYZ microscope objective"
              n93 = case shown="True" "KCube Shutter On?" {
                frame False {
                }
                frame True {
                  n94 = local read "KCubeSolenoidControl"() -> (w135:refnum<k24>)
                  n95 = property class="KCubeSolenoidControl"(reference=w135, "SerialNumber"="68001425") -> (reference out=w133:refnum<k24>)  [unwired: 1 in, 1 out]
                  n96 = invoke class="KCubeSolenoidControl" method="CreateDevice"(reference=w133) -> (reference out=w132:refnum<k24>)  [unwired: 2 in, 2 out]
                  n97 = property class="KCubeSolenoidControl"(reference=w132) -> (reference out=w131:refnum<k24>, "Device"=w130:refnum<k24>)  [unwired: 1 in, 1 out]
                  n98 = local read "Log file"() -> (w127:string)
                  n99 = local write "KCubeSolenoidControl Reference"(w131) -> ()
                  n100 = invoke class="KCubeSolenoid" method="GetOperatingState"(reference=w130) -> (reference out=w129:refnum<k24>, "GetOperatingState"=w128:i32)  [unwired: 2 in, 1 out]
                  n101 = local write "KCube Shutter Device Reference"(w129) -> ()
                  n102 = call "Write2LogFile.vi"("Add to log file"="Initialise communication with Shutter", "Log file before"=w127) -> ("Log file after"=w126:string)
                  n103 = case shown="2, Default" w128 {
                    frame 1 {
                      n104 = property on="Shutter Ctrls" class="Ring (strict)"("Value"=u16 5 ("Shutter Ctrls")) -> ()  [unwired: 2 in, 2 out]
                    }
                    frame 2, Default {
                      n105 = property on="Shutter Ctrls" class="Ring (strict)"("Value"=u16 0 ("Shutter Ctrls")) -> ()  [unwired: 2 in, 2 out]
                    }
                  }
                  n106 = local write "Log file"(w126) -> ()
                }
              }
              n107 = case shown="True" "KCubes Piezo On?" {
                frame False {
                }
                frame True {
                  # "Initialise microscope objective XYZ piezo and solenoid shutter devices"
                  n108 = local read "KCubePiezoControl Z"() -> (w158:refnum<k24>)
                  n109 = local read "KCubePiezoControl X"() -> (w152:refnum<k24>)
                  n110 = local read "KCubePiezoControl Y"() -> (w151:refnum<k24>)
                  n111 = property class="KCubePiezoControl"(reference=w158, "SerialNumber"="29502682") -> (reference out=w156:refnum<k24>)  [unwired: 1 in, 1 out]
                  n112 = property class="KCubePiezoControl"(reference=w151, "SerialNumber"="29502721") -> (reference out=w147:refnum<k24>)  [unwired: 1 in, 1 out]
                  n113 = property class="KCubePiezoControl"(reference=w152, "SerialNumber"="29250034") -> (reference out=w148:refnum<k24>)  [unwired: 1 in, 1 out]
                  n114 = local read "Log file"() -> (w140:string)
                  n115 = call "Write2LogFile.vi"("Add to log file"="Initialise communication with Piezos", "Log file before"=w140) -> ("Log file after"=w139:string)
                  n116 = local write "Log file"(w139) -> ()
                  n117 = invoke class="KCubePiezoControl" method="CreateDevice"(reference=w156) -> (reference out=w155:refnum<k24>)  [unwired: 2 in, 2 out]
                  n118 = invoke class="KCubePiezoControl" method="CreateDevice"(reference=w147) -> (reference out=w146:refnum<k24>)  [unwired: 2 in, 2 out]
                  n119 = invoke class="KCubePiezoControl" method="CreateDevice"(reference=w148) -> (reference out=w145:refnum<k24>)  [unwired: 2 in, 2 out]
                  n120 = property class="KCubePiezoControl"(reference=w155) -> (reference out=w154:refnum<k24>, "Device"=w153:refnum<k24>)  [unwired: 1 in, 1 out]
                  n121 = property class="KCubePiezoControl"(reference=w145) -> (reference out=w142:refnum<k24>, "Device"=w141:refnum<k24>)  [unwired: 1 in, 1 out]
                  n122 = local write "KCubePiezoControl Z Reference"(w154) -> ()
                  n123 = local write "KCubePiezoDevice Z Reference"(w153) -> ()
                  n124 = local write "KCubePiezoControl X Reference"(w142) -> ()
                  n125 = local write "KCubePiezoDevice X Reference"(w141) -> ()
                  n126 = property class="KCubePiezoControl"(reference=w146) -> (reference out=w144:refnum<k24>, "Device"=w143:refnum<k24>)  [unwired: 1 in, 1 out]
                  n127 = local write "KCubePiezoControl Y Reference"(w144) -> ()
                  n128 = local write "KCubePiezoDevice Y Reference"(w143) -> ()
                }
              }
            }
            frame #6 {
              # "ESP 300: 1 Jobin Yvon 320 Monochromator"
              n129 = case shown="True" "ESP 300 On?" {
                frame False {
                }
                frame True {
                  w168 = 1 ("Axis")
                  # "Initialise communication with ESP300"
                  n130 = local read "ESP 300 COM Port"() -> (w173:refnum<visa-resource-name>)
                  n131 = local read "ESP300 Error"() -> (w172:errorcluster)
                  n132 = local read "Log file"() -> (w162:string)
                  n133 = call "Write2LogFile.vi"("Add to log file"="Initialise communication with ESP 300", "Log file before"=w162) -> ("Log file after"=w161:string)
                  n134 = call "Init Communication.vi"("error in (no error)"=w172, "VISA resource name in"=w173) -> ("error out"=w170:errorcluster, "VISA resource name out"=w171:refnum<visa-resource-name>)  [unwired: 8 in]
                  n135 = local write "Log file"(w161) -> ()
                  n136 = call "QMotor On.vi"("error in (no error)"=w170, "Axis"=w168, "VISA resource name in"=w171) -> ("error out"=w167:errorcluster, "Motor On?"=w169:bool, "VISA resource name out"=w164:refnum<visa-resource-name>)  [unwired: 6 in]
                  n137 = local write "Mono2 On"(w169) -> ()
                  n138 = call "QPosition.vi"("error in (no error)"=w167, "Axis"=w168, "VISA resource name in"=w164) -> ("error out"=w166:errorcluster, "Position"=w163:dbl, "VISA resource name out"=w165:refnum<visa-resource-name>)  [unwired: 6 in]
                  n139 = local write "ESP 300 COM Port"(w165) -> ()
                  n140 = local write "Mono2 Motor Position"(w163) -> ()
                  n141 = local write "ESP300 Error"(w166) -> ()
                }
              }
            }
            frame #7 {
              # "448.3nm Laser Diode + Temp Controller & Driver"
              n142 = case shown="True" "Laser Comm On?" {
                frame False {
                }
                frame True {
                  n143 = disable-structure shown="Disabled" {
                    frame Disabled {
                      n144 = control-ref of="This VI"() -> (w203:refnum<vi>)
                      n145 = call <instrlib>:"z_ConnectToTL4000-Device.vi"("VI reference"=w203, "Models"=string[] ["CLD1"], "Manufacturer"="Thorlabs") -> ()  [unwired: 6 in, 3 out]
                    }
                    frame Enabled {
                    }
                  }
                  n146 = local read "Diode Driver Error"() -> (w182:errorcluster)
                  n147 = call <instrlib>:"TL4000 Initialize.vi"("error in (no error)"=w182, "resource name"=refnum<visa-resource-name> "USB0::0x1313::0x804F::M00549740::INSTR" ("Diode Driver COM")) -> ("error out"=w190:errorcluster, "instrument handle out"=w191:refnum<visa-resource-name>)  [unwired: 8 in]
                  n148 = call <instrlib>:"TL4000 Identification Query.vi"("error in (no error)"=w190, "instrument handle"=w191) -> ("error out"=w186:errorcluster, "instrument handle out"=w188:refnum<visa-resource-name>, "Serial Number"=→"Serial Number":string)  [unwired: 4 in, 3 out]
                  n149 = local read "Laser Diode Current Set"() -> (w193:dbl)
                  n150 = call <instrlib>:"TL4000 Beep.vi"("error in (no error)"=w186, "instrument handle"=w188) -> ("error out"=w185:errorcluster, "instrument handle out"=w187:refnum<visa-resource-name>)  [unwired: 8 in]
                  n151 = call <instrlib>:"TL4000 Get TEC Output State.vi"("error in (no error)"=w185, "instrument handle"=w187) -> ("error out"=w201:errorcluster, "TEC Output"=w180:bool, "instrument handle out"=w200:refnum<visa-resource-name>)  [unwired: 7 in]
                  n152 = property on="Laser Safety" class="Ring (strict)"("Visible"=w180) -> ()  [unwired: 2 in, 2 out]
                  n153 = property on="Laser on? Control" class="Bool (strict)"("Visible"=w180) -> ()  [unwired: 2 in, 2 out]
                  n154 = Not(x=w180) -> (.not. x?=w196:bool)
                  n155 = local write "TEC Output"(w180) -> ()
                  n156 = call <instrlib>:"TL4000 Get LD Output State.vi"("error in (no error)"=w201, "instrument handle"=w200) -> ("error out"=w197:errorcluster, "LD Output"=w202:bool, "instrument handle out"=w198:refnum<visa-resource-name>)  [unwired: 7 in]
                  n157 = local write "Laser on?"(w202) -> ()
                  n158 = call <instrlib>:"TL4000 Measure Temperature.vi"("error in (no error)"=w197, "instrument handle"=w198) -> ("error out"=w194:errorcluster, "Temperature"=→"TEC Temperature":dbl, "instrument handle out"=w195:refnum<visa-resource-name>)  [unwired: 7 in]
                  n159 = property on="TEC Output" class="Bool (strict)"("Visible"=w196) -> ()  [unwired: 2 in, 2 out]
                  n160 = call <instrlib>:"TL4000 Set Laser Diode Current Setpoint.vi"("error in (no error)"=w194, "Laser Diode Current Setpoint (0.0)"=w193, "instrument handle"=w195) -> ("error out"=w179:errorcluster, "instrument handle out"=w178:refnum<visa-resource-name>)  [unwired: 7 in]
                  n161 = call <instrlib>:"TL4000 Set Laser Diode Current Limit.vi"("error in (no error)"=w179, "Laser Diode Current Limit (0.0)"=0.061, "instrument handle"=w178) -> ("error out"=w176:errorcluster, "instrument handle out"=w177:refnum<visa-resource-name>)  [unwired: 7 in]
                  n162 = call <instrlib>:"TL4000 Set Temperature Setpoint.vi"("error in (no error)"=w176, "Temperature Setpoint (25.0)"=25.0, "instrument handle"=w177) -> ("error out"=w184:errorcluster, "instrument handle out"=w183:refnum<visa-resource-name>)  [unwired: 7 in]
                  n163 = local write "Diode Driver COM"(w183) -> ()
                  n164 = local write "Diode Driver Error"(w184) -> ()
                }
              }
            }
            frame #8 {
              # "Visualisation camera?"
              n165 = call "uc480_SubVI_Example_CameraInit.vi"("Camera ID"=0, "Init Camera Flag"=TRUE) -> ("Error Out"=w206:errorcluster, ".NET (Reference)"=w207:refnum<k24>)  [unwired: 8 in]
              n166 = local write "Thorcam Error"(w206) -> ()
              n167 = local write "ThorCam Reference"(w207) -> ()
            }
            frame #9 {
              # "Final activation message"
            }
          }
        }
      }
      n168 = local read "Log file"() -> (w9:string)
      n169 = call "Write2LogFile.vi"("Add to log file"=w8, "Log file before"=w9) -> ("Log file after"=w7:string)
      n170 = local write "Log file"(w7) -> ()
    }
    frame #1 {
      # "Main Program"
      n171 = while {
        stop <- w211 stop-if-true
        n172 = event shown="[19] \"ThorCam Init\": Mouse Down" {
          selector: _ -> [_ _ _ _ _ _ _ _ _ _ _ _ _ _ _ _ _ _ _ _ _ _ _ _ _ _ _ _ _]
          dyn-events: _ -> [_ _ _ _ _ _ _ _ _ _ _ _ _ _ _ _ _ _ _ _ _ _ _ _ _ _ _ _ _]
          timeout: _ -> [_ _ _ _ _ _ _ _ _ _ _ _ _ _ _ _ _ _ _ _ _ _ _ _ _ _ _ _ _]
          tunnel: [w212 _ _ _ _ _ _ _ _ _ _ _ _ _ _ _ _ _ _ _ _ _ _ _ _ _ _ _ _] -> w211
          event "Stop Everything & Quit?": Value Change {
            n173 = event-data() -> ("NewVal"=w212:bool)  [unwired: 1 in, 5 out]
          }
          event Value Change {
            n174 = event-data() -> ()  [unwired: 1 in, 6 out]
            n175 = local read "Acq Mode"() -> (w213:T2)
            n176 = case shown="\"Spectrum\"" w213 {
              frame "Image" {
                w215 = TRUE
                w216 = FALSE
                n177 = property on="Exit mirror" class="Enum (strict)"("Val(Sgnl)"=enum16{"CCD", "APD"}."CCD" ("Exit mirror")) -> ()  [unwired: 2 in, 2 out]
                n178 = property on="Background substract" class="Enum (strict)"("Visible"=w215) -> ()  [unwired: 2 in, 2 out]
                n179 = property on="CCD ROI" class="Enum (strict)"("Visible"=w215) -> ()  [unwired: 2 in, 2 out]
                n180 = property on="Accumulations" class="DigNum (strict)"("Visible"=w215) -> ()  [unwired: 2 in, 2 out]
                n181 = property on="CCD 2D Image Main" class="IntGraph (strict)"("Visible"=w215) -> ()  [unwired: 2 in, 2 out]
                n182 = property on="CCD 2D Image XY Map" class="IntGraph (strict)"("Visible"=w215) -> ()  [unwired: 2 in, 2 out]
                n183 = property on="Exposure Time (ms)" class="DigNum (strict)"("Visible"=w215) -> ()  [unwired: 2 in, 2 out]
                n184 = property on="CCD 1D Spectrum XY Map" class="WFGraph (strict)"("Visible"=w216) -> ()  [unwired: 2 in, 2 out]
                n185 = property on="CCD 1D Spectrum Main" class="XYGraph (strict)"("Visible"=w216) -> ()  [unwired: 2 in, 2 out]
              }
              frame "Spectrum" {
                w219 = FALSE
                w218 = TRUE
                n186 = property on="CCD 2D Image XY Map" class="IntGraph (strict)"("Visible"=w219) -> ()  [unwired: 2 in, 2 out]
                n187 = property on="CCD 2D Image Main" class="IntGraph (strict)"("Visible"=w219) -> ()  [unwired: 2 in, 2 out]
                n188 = property on="Background substract" class="Enum (strict)"("Visible"=w218) -> ()  [unwired: 2 in, 2 out]
                n189 = property on="CCD ROI" class="Enum (strict)"("Visible"=w218) -> ()  [unwired: 2 in, 2 out]
                n190 = property on="Accumulations" class="DigNum (strict)"("Visible"=w218) -> ()  [unwired: 2 in, 2 out]
                n191 = property on="CCD 1D Spectrum XY Map" class="WFGraph (strict)"("Visible"=w218) -> ()  [unwired: 2 in, 2 out]
                n192 = property on="Exposure Time (ms)" class="DigNum (strict)"("Visible"=w218) -> ()  [unwired: 2 in, 2 out]
                n193 = property on="CCD 1D Spectrum Main" class="XYGraph (strict)"("Visible"=w218) -> ()  [unwired: 2 in, 2 out]
                n194 = property on="Exit mirror" class="Enum (strict)"("Val(Sgnl)"=enum16{"CCD", "APD"}."CCD" ("Exit mirror")) -> ()  [unwired: 2 in, 2 out]
              }
              frame "APD 1" {
                w221 = FALSE
                w222 = TRUE
                n195 = property on="Exit mirror" class="Enum (strict)"("Val(Sgnl)"=enum16{"CCD", "APD"}."APD" ("Exit mirror")) -> ()  [unwired: 2 in, 2 out]
                n196 = property on="Background substract" class="Enum (strict)"("Visible"=w221) -> ()  [unwired: 2 in, 2 out]
                n197 = property on="CCD ROI" class="Enum (strict)"("Visible"=w221) -> ()  [unwired: 2 in, 2 out]
                n198 = property on="Accumulations" class="DigNum (strict)"("Visible"=w221) -> ()  [unwired: 2 in, 2 out]
                n199 = property on="CCD 2D Image Main" class="IntGraph (strict)"("Visible"=w221) -> ()  [unwired: 2 in, 2 out]
                n200 = property on="CCD 2D Image XY Map" class="IntGraph (strict)"("Visible"=w221) -> ()  [unwired: 2 in, 2 out]
                n201 = property on="Exposure Time (ms)" class="DigNum (strict)"("Visible"=w221) -> ()  [unwired: 2 in, 2 out]
                n202 = property on="CCD 1D Spectrum XY Map" class="WFGraph (strict)"("Visible"=w222) -> ()  [unwired: 2 in, 2 out]
                n203 = property on="CCD 1D Spectrum Main" class="XYGraph (strict)"("Visible"=w222) -> ()  [unwired: 2 in, 2 out]
              }
              frame "APD 2" {
                w224 = FALSE
                w225 = TRUE
                n204 = property on="Exit mirror" class="Enum (strict)"("Val(Sgnl)"=enum16{"CCD", "APD"}."APD" ("Exit mirror")) -> ()  [unwired: 2 in, 2 out]
                n205 = property on="Background substract" class="Enum (strict)"("Visible"=w224) -> ()  [unwired: 2 in, 2 out]
                n206 = property on="CCD ROI" class="Enum (strict)"("Visible"=w224) -> ()  [unwired: 2 in, 2 out]
                n207 = property on="Accumulations" class="DigNum (strict)"("Visible"=w224) -> ()  [unwired: 2 in, 2 out]
                n208 = property on="CCD 2D Image Main" class="IntGraph (strict)"("Visible"=w224) -> ()  [unwired: 2 in, 2 out]
                n209 = property on="CCD 2D Image XY Map" class="IntGraph (strict)"("Visible"=w224) -> ()  [unwired: 2 in, 2 out]
                n210 = property on="Exposure Time (ms)" class="DigNum (strict)"("Visible"=w224) -> ()  [unwired: 2 in, 2 out]
                n211 = property on="CCD 1D Spectrum XY Map" class="WFGraph (strict)"("Visible"=w225) -> ()  [unwired: 2 in, 2 out]
                n212 = property on="CCD 1D Spectrum Main" class="XYGraph (strict)"("Visible"=w225) -> ()  [unwired: 2 in, 2 out]
              }
              frame "APD 1+2" {
                w227 = FALSE
                w228 = TRUE
                n213 = property on="Exit mirror" class="Enum (strict)"("Val(Sgnl)"=enum16{"CCD", "APD"}."APD" ("Exit mirror")) -> ()  [unwired: 2 in, 2 out]
                n214 = property on="Background substract" class="Enum (strict)"("Visible"=w227) -> ()  [unwired: 2 in, 2 out]
                n215 = property on="Accumulations" class="DigNum (strict)"("Visible"=w227) -> ()  [unwired: 2 in, 2 out]
                n216 = property on="CCD ROI" class="Enum (strict)"("Visible"=w227) -> ()  [unwired: 2 in, 2 out]
                n217 = property on="CCD 2D Image Main" class="IntGraph (strict)"("Visible"=w227) -> ()  [unwired: 2 in, 2 out]
                n218 = property on="CCD 2D Image XY Map" class="IntGraph (strict)"("Visible"=w227) -> ()  [unwired: 2 in, 2 out]
                n219 = property on="Exposure Time (ms)" class="DigNum (strict)"("Visible"=w227) -> ()  [unwired: 2 in, 2 out]
                n220 = property on="CCD 1D Spectrum XY Map" class="WFGraph (strict)"("Visible"=w228) -> ()  [unwired: 2 in, 2 out]
                n221 = property on="CCD 1D Spectrum Main" class="XYGraph (strict)"("Visible"=w228) -> ()  [unwired: 2 in, 2 out]
              }
            }
          }
          event "FSM X Axis Pos", "FSM Y Axis Pos": Value Change {
            w230 = 10.0 ("maximum value")
            n222 = event-data() -> ("CtlRef"=w235:refnum<vi>, "NewVal"=w231:dbl)  [unwired: 1 in, 4 out]
            n223 = property class="DigNum (strict)"(reference=w235) -> ("Label.Text"=w234:string)  [unwired: 1 in, 2 out]
            n224 = case shown="\"FSM X Axis Pos\", Default" w234 {
              tunnel: [w236 w237] -> w229
              frame "FSM Y Axis Pos" {
                n225 = local read "FSM Y Axis"() -> (w236:tag)
              }
              frame "FSM X Axis Pos", Default {
                n226 = local read "FSM X Axis"() -> (w237:tag)
              }
            }
            n227 = Negate(x=w230) -> (-x=w232:dbl)
            n228 = call-poly <vilib>:"DAQmx Create Virtual Channel.vi"("maximum value"=w230, "minimum value"=w232, "physical channels"=w229) -> ("task out"=w233:refnum<k21>)  [unwired: 11 in, 1 out]
            n229 = call-poly <vilib>:"DAQmx Write.vi"("task/channels in"=w233, "data"=w231) -> ()  [unwired: 11 in, 3 out]
          }
          event "FSM Up", "FSM Down", "FSM Left", "FSM Right": Mouse Down {
            w244 = 10.0 ("maximum value")
            n230 = event-data() -> ("CtlRef"=w239:refnum<vi>)  [unwired: 1 in, 5 out]
            n231 = property class="Bool (strict)"(reference=w239) -> ("Label.Text"=w238:string)  [unwired: 1 in, 2 out]
            n232 = local read "FSM Axis Step"() -> (w242:dbl)
            n233 = case shown="\"FSM Right\"" w238 {
              tunnel: [w249 w253 w257 w261] -> w245
              tunnel: w242 -> [w247 w251 w255 w259]
              tunnel: [w246 w250 w254 w258] -> w241
              frame "FSM Up", Default {
                n234 = local read "FSM Y Axis Pos"() -> (w248:dbl)
                n235 = Add(x=w248, y=w247) -> (x+y=w246:dbl)
                n236 = local write "FSM Y Axis Pos"(w246) -> ()
                n237 = local read "FSM Y Axis"() -> (w249:tag)
              }
              frame "FSM Down" {
                n238 = local read "FSM Y Axis Pos"() -> (w252:dbl)
                n239 = Subtract(x=w252, y=w251) -> (x-y=w250:dbl)
                n240 = local write "FSM Y Axis Pos"(w250) -> ()
                n241 = local read "FSM Y Axis"() -> (w253:tag)
              }
              frame "FSM Left" {
                n242 = local read "FSM X Axis Pos"() -> (w256:dbl)
                n243 = Subtract(x=w256, y=w255) -> (x-y=w254:dbl)
                n244 = local write "FSM X Axis Pos"(w254) -> ()
                n245 = local read "FSM X Axis"() -> (w257:tag)
              }
              frame "FSM Right" {
                n246 = local read "FSM X Axis Pos"() -> (w260:dbl)
                n247 = Add(x=w260, y=w259) -> (x+y=w258:dbl)
                n248 = local write "FSM X Axis Pos"(w258) -> ()
                n249 = local read "FSM X Axis"() -> (w261:tag)
              }
            }
            n250 = Negate(x=w244) -> (-x=w243:dbl)
            n251 = call-poly <vilib>:"DAQmx Create Virtual Channel.vi"("maximum value"=w244, "minimum value"=w243, "physical channels"=w245) -> ("task out"=w240:refnum<k21>)  [unwired: 11 in, 1 out]
            n252 = call-poly <vilib>:"DAQmx Write.vi"("task/channels in"=w240, "data"=w241) -> ()  [unwired: 11 in, 3 out]
          }
          event "Conv/Energy (eV)", "Conv/Wavelength (nm)", "Conv/Time (s)", "Conv/Wavenumber (m-1)": Value Change {
            n253 = event-data() -> ("CtlRef"=w264:refnum<vi>, "NewVal"=w262:dbl)  [unwired: 1 in, 4 out]
            n254 = property class="DigNum (strict)"(reference=w264) -> ("Label.Text"=w263:string)  [unwired: 1 in, 2 out]
            n255 = case shown="\"Conv/Wavenumber (m-1)\"" w263 {
              tunnel: w262 -> [w272 _ w285 _]
              frame "Conv/Wavelength (nm)", Default {
                n256 = Multiply(x=w272, y=1e-09) -> (x*y=w270:dbl)
                n257 = Divide(x=1.0, y=w270) -> (x/y=w267:dbl)
                n258 = Divide(x=w270, y=299792458.0) -> (x/y=w269:dbl)
                n259 = Divide(x=w267, y=100.0) -> (x/y=w265:dbl)
                n260 = Divide(x=1239.841, y=w272) -> (x/y=w274:dbl)
                n261 = local write "Conv/Energy (eV)"(w274) -> ()
                n262 = local write "Conv/Wavenumber (m-1)"(w265) -> ()
                n263 = local write "Conv/Time (s)"(w269) -> ()
              }
              frame "Conv/Time (s)" {
              }
              frame "Conv/Energy (eV)" {
                n264 = Divide(x=1239.841, y=w285) -> (x/y=w284:dbl)
                n265 = Multiply(x=w284, y=1e-09) -> (x*y=w281:dbl)
                n266 = local write "Conv/Wavelength (nm)"(w284) -> ()
                n267 = Divide(x=1.0, y=w281) -> (x/y=w278:dbl)
                n268 = Divide(x=w278, y=100.0) -> (x/y=w276:dbl)
                n269 = Divide(x=w281, y=299792458.0) -> (x/y=w279:dbl)
                n270 = local write "Conv/Wavenumber (m-1)"(w276) -> ()
                n271 = local write "Conv/Time (s)"(w279) -> ()
              }
              frame "Conv/Wavenumber (m-1)" {
              }
            }
          }
          event "FSM Home": Mouse Down {
            w291 = 0.0 ("FSM X Axis Pos")
            w292 = 0.0 ("FSM X Axis Pos")
            n272 = event-data() -> ()  [unwired: 1 in, 6 out]
            n273 = local read "FSM X Axis"() -> (w293:tag)
            n274 = local read "FSM Y Axis"() -> (w290:tag)
            n275 = Negate(x=10.0 ("maximum value")) -> (-x=w287:dbl)
            n276 = Negate(x=10.0 ("maximum value")) -> (-x=w296:dbl)
            n277 = call-poly <vilib>:"DAQmx Create Virtual Channel.vi"("minimum value"=w287, "physical channels"=w290) -> ("task out"=w289:refnum<k21>)  [unwired: 12 in, 1 out]
            n278 = call-poly <vilib>:"DAQmx Create Virtual Channel.vi"("minimum value"=w296, "physical channels"=w293) -> ("task out"=w294:refnum<k21>)  [unwired: 12 in, 1 out]
            n279 = local write "FSM Y Axis Pos"(w291) -> ()
            n280 = local write "FSM X Axis Pos"(w292) -> ()
            n281 = call-poly <vilib>:"DAQmx Write.vi"("task/channels in"=w289, "data"=w291) -> ()  [unwired: 11 in, 3 out]
            n282 = call-poly <vilib>:"DAQmx Write.vi"("task/channels in"=w294, "data"=w292) -> ()  [unwired: 11 in, 3 out]
          }
          event "Exit mirror": Value Change {
            n283 = event-data() -> ("NewVal"=w298:enum16{"CCD", "APD"})  [unwired: 1 in, 5 out]
            n284 = case shown="\"CCD\"" w298 {
              tunnel: ["uPL" w331] -> w301
              tunnel: [TRUE FALSE] -> w300
              tunnel: ["CCD" w331] -> w297
              frame "CCD" {
                # "mono + CCD"
              }
              frame "APD" {
                w331 = "APD"
                # "mono only\nAPD exit port"
              }
            }
            n285 = local read "LightField Automation error out"() -> (w304:errorcluster)
            n286 = local read "LightField Automation out"() -> (w305:refnum<class "LightField Automation.lvclass">)
            n287 = stacked-sequence {
              seq-local: [w314 _ _] -> [_ w320 _]
              seq-local: [w313 _ _] -> [_ w319 _]
              seq-local: [w312 _ _] -> [_ w316 _]
              seq-local: [w311 _ _] -> [_ w315 _]
              seq-local: [_ w318 _] -> [_ _ w327]
              seq-local: [_ w317 _] -> [_ _ w326]
              seq-local: [_ w315 _] -> [_ _ w323]
              tunnel: w305 -> [w314 _ _]
              tunnel: w304 -> [w313 _ _]
              tunnel: w301 -> [w312 _ _]
              tunnel: w297 -> [w311 _ _]
              tunnel: [_ _ w327] -> w303
              tunnel: [_ _ w326] -> w302
              frame #0 {
                n288 = local read "Log file"() -> (w309:string)
                n289 = call "Write2LogFile.vi"("Add to log file"="Changing SpectraPro HRS-500 exit port ...", "Log file before"=w309) -> ("Log file after"=w310:string)
                n290 = local write "Log file"(w310) -> ()
              }
              frame #1 {
                n291 = call "Exp_SetExperiment.vi"("error in (no error)"=w319, "ExperimentName"=w316, "LightField Automation in"=w320) -> ("error out"=w318:errorcluster, "LightField Automation out"=w317:refnum<class "LightField Automation.lvclass">)  [unwired: 7 in]
              }
              frame #2 {
                n292 = local read "Log file"() -> (w325:string)
                n293 = Concatenate Strings("SpectraPro HRS-500 exit mirror set to " ("string"), w323) -> (w321:string)
                n294 = call "Write2LogFile.vi"("Add to log file"=w321, "Log file before"=w325) -> ("Log file after"=w324:string)
                n295 = local write "Log file"(w324) -> ()
              }
            }
            n296 = property on="Exposure Time (ms)" class="DigNum (strict)"("Visible"=w300) -> ()  [unwired: 2 in, 2 out]
            n297 = call "spec_GetOpticalExitPort.vi"("error in (no error)"=w303, "LightField Automation in"=w302) -> ("error out"=w306:errorcluster, "Exit Port Location"=→"Exit Port Location":T6, "LightField Automation out"=w307:refnum<class "LightField Automation.lvclass">)  [unwired: 7 in]
            n298 = local write "LightField Automation out"(w307) -> ()
            n299 = local write "LightField Automation error out"(w306) -> ()
          }
          event "Mono2 On": Value Change {
            n300 = event-data() -> ("NewVal"=w333:bool)  [unwired: 1 in, 5 out]
            n301 = case shown="True" w333 {
              frame False {
                n302 = stacked-sequence {
                  frame #0 {
                    n303 = local read "ESP 300 COM Port"() -> (w337:refnum<visa-resource-name>)
                    n304 = local read "ESP300 Error"() -> (w338:errorcluster)
                    n305 = call "Motor Off.vi"("error in (no error)"=w338, "Axis"=1, "VISA resource name in"=w337) -> ("error out"=w335:errorcluster, "VISA resource name out"=w334:refnum<visa-resource-name>)  [unwired: 7 in]
                    n306 = local write "ESP 300 COM Port"(w334) -> ()
                    n307 = local write "ESP300 Error"(w335) -> ()
                  }
                  frame #1 {
                    n308 = local read "Log file"() -> (w340:string)
                    n309 = call "Write2LogFile.vi"("Add to log file"="Mono2 motor turned off", "Log file before"=w340) -> ("Log file after"=w341:string)
                    n310 = local write "Log file"(w341) -> ()
                  }
                }
              }
              frame True {
                n311 = stacked-sequence {
                  frame #0 {
                    n312 = local read "ESP 300 COM Port"() -> (w345:refnum<visa-resource-name>)
                    n313 = local read "ESP300 Error"() -> (w346:errorcluster)
                    n314 = call "Motor On.vi"("error in (no error)"=w346, "Axis"=1, "VISA resource name in"=w345) -> ("error out"=w343:errorcluster, "VISA resource name out"=w342:refnum<visa-resource-name>)  [unwired: 7 in]
                    n315 = local write "ESP 300 COM Port"(w342) -> ()
                    n316 = local write "ESP300 Error"(w343) -> ()
                  }
                  frame #1 {
                    n317 = local read "Log file"() -> (w348:string)
                    n318 = call "Write2LogFile.vi"("Add to log file"="Mono2 motor turned on", "Log file before"=w348) -> ("Log file after"=w349:string)
                    n319 = local write "Log file"(w349) -> ()
                  }
                }
              }
            }
          }
          event "Excitation Power (uW)": Mouse Down; "Excitation Wavelength (nm)": Value Change {
            n320 = event-data() -> ()  [unwired: 1 in, 4 out]
            n321 = local read "Excitation Wavelength (nm)"() -> (w356:dbl)
            n322 = local read "Photodiode handle out"() -> (w357:refnum<visa-resource-name>)
            n323 = local read "Photodiode error out"() -> (w355:errorcluster)
            n324 = call <instrlib>:"TLPM Set Wavelength.vi"("error in (no error)"=w355, "Wavelength (0.0)"=w356, "instrument handle"=w357) -> ("error out"=w354:errorcluster, "instrument handle out"=w353:refnum<visa-resource-name>)  [unwired: 7 in]
            n325 = call <instrlib>:"TLPM Measure Power.vi"("error in (no error)"=w354, "instrument handle"=w353) -> ("error out"=w350:errorcluster, "Power"=w352:dbl, "instrument handle out"=w351:refnum<visa-resource-name>)  [unwired: 7 in]
            n326 = local write "Photodiode handle out"(w351) -> ()
            n327 = local write "Excitation Power (uW)"(w352) -> ()
            n328 = local write "Photodiode error out"(w350) -> ()
          }
          event "CCD 1D Spectrum Main", "Polarisation 1D Spectrum": Scale Range Change {
            n329 = event-data() -> ("CtlRef"=w359:refnum<vi>, "ScaleRef"=w361:refnum<vi>, "NewRange"=w358:T10)  [unwired: 1 in, 5 out]
            n330 = property class="GrphScl"(reference=w361) -> ("NameLbl.Text"=w360:string)  [unwired: 1 in, 2 out]
            n331 = case shown="\"Energy (eV)\"" w360 {
              tunnel: w359 -> [w364 _]
              tunnel: w358 -> [w362 _]
              frame "Energy (eV)" {
                w363 = 1239.841
                n332 = property class="XYGraph (strict)"(reference=w364) -> ("Label.Text"=w369:string)  [unwired: 1 in, 2 out]
                n333 = Unbundle By Name(w362) -> ("Minimum"=w366:dbl, "Maximum"=w365:dbl)
                n334 = Divide(x=w363, y=w366) -> (x/y=w367:dbl)
                n335 = Divide(x=w363, y=w365) -> (x/y=w368:dbl)
                n336 = case shown="\"Polarisation 1D Spectrum\"" w369 {
                  tunnel: w367 -> [w371 w373]
                  tunnel: w368 -> [w370 w372]
                  frame "CCD 1D Spectrum Main", Default {
                    n337 = property on="CCD 1D Spectrum Main Energy Scale" class="XYGraph (strict)"("XScale.Maximum"=w371, "XScale.Minimum"=w370) -> ()  [unwired: 2 in, 2 out]
                  }
                  frame "Polarisation 1D Spectrum" {
                    n338 = property on="Polarisation 1D Spectrum Energy Scale" class="XYGraph (strict)"("XScale.Maximum"=w373, "XScale.Minimum"=w372) -> ()  [unwired: 2 in, 2 out]
                  }
                }
              }
              frame "PL Intensity (cts)", Default {
              }
            }
          }
          event "Full scale": Mouse Down {
            w378 = 1239.84
            n339 = event-data() -> ()  [unwired: 1 in, 8 out]
            n340 = property on="CCD 1D Spectrum Main" class="XYGraph (strict)"("XScale.ScaleFit"=u8 1 ("X Scale.Scale Fit")) -> ("XScale.Minimum"=w377:dbl, "XScale.Maximum"=w376:dbl)  [unwired: 2 in, 2 out]
            n341 = Divide(x=w378, y=w377) -> (x/y=w375:dbl)
            n342 = Divide(x=w378, y=w376) -> (x/y=w374:dbl)
            n343 = property on="CCD 1D Spectrum Main Energy Scale" class="XYGraph (strict)"("XScale.Maximum"=w375, "XScale.Minimum"=w374) -> ()  [unwired: 2 in, 2 out]
          }
          event "Grating": Value Change {
            n344 = event-data() -> ("NewVal"=w388:string)  [unwired: 1 in, 5 out]
            n345 = local read "LightField Automation error out"() -> (w389:errorcluster)
            n346 = local read "LightField Automation out"() -> (w390:refnum<class "LightField Automation.lvclass">)
            n347 = stacked-sequence {
              seq-local: [w396 _ _] -> [_ w401 _]
              seq-local: [w395 _ _] -> [_ w400 _]
              seq-local: [w394 _ _] -> [_ w397 _]
              seq-local: [_ w399 _] -> [_ _ w408]
              seq-local: [_ w398 _] -> [_ _ w407]
              seq-local: [_ w397 _] -> [_ _ w405]
              tunnel: w390 -> [w396 _ _]
              tunnel: w389 -> [w395 _ _]
              tunnel: w388 -> [w394 _ _]
              tunnel: [_ _ w408] -> w384
              tunnel: [_ _ w407] -> w383
              frame #0 {
                n348 = local read "Log file"() -> (w392:string)
                n349 = call "Write2LogFile.vi"("Add to log file"="Changing grating ...", "Log file before"=w392) -> ("Log file after"=w393:string)
                n350 = local write "Log file"(w393) -> ()
              }
              frame #1 {
                n351 = call "spec_SetGrating.vi"("error in (no error)"=w400, "GratingSelected"=w397, "LightField Automation in"=w401) -> ("error out"=w398:errorcluster, "LightField Automation out"=w399:refnum<class "LightField Automation.lvclass">)  [unwired: 7 in]
              }
              frame #2 {
                n352 = local read "Log file"() -> (w404:string)
                n353 = Concatenate Strings("Grating changed to " ("string"), w405) -> (w403:string)
                n354 = call "Write2LogFile.vi"("Add to log file"=w403, "Log file before"=w404) -> ("Log file after"=w402:string)
                n355 = local write "Log file"(w402) -> ()
              }
            }
            n356 = call "spec_GetCenterWavelength.vi"("error in (no error)"=w383, "LightField Automation in"=w384) -> ("error out"=w382:errorcluster, "Center Wavelength"=w380:dbl, "LightField Automation out"=w381:refnum<class "LightField Automation.lvclass">)  [unwired: 7 in]
            n357 = local write "Center Wavelength (nm)"(w380) -> ()
            n358 = call "spec_getCalibration.vi"("error in (no error)"=w382, "LightField Automation in"=w381) -> ("error out"=w386:errorcluster, "ColumnCalibration"=w385:dbl[], "LightField Automation out"=w387:refnum<class "LightField Automation.lvclass">)  [unwired: 7 in]
            n359 = local write "LightField Automation out"(w387) -> ()
            n360 = local write "Wavelength calibration"(w385) -> ()
            n361 = local write "LightField Automation error out"(w386) -> ()
          }
          event "Acquire Spectrum", "Acquire Continuous Spectrum", "Acquire Polarisation", "Acquire XY Map": Mouse Down {
            n362 = event-data() -> ("CtlRef"=w409:refnum<vi>)  [unwired: 1 in, 6 out]
            n363 = stacked-sequence {
              tunnel: w409 -> [w410 w537]
              frame #0 {
                # "Actual measurements"
                n364 = local read "LightField Automation error out"() -> (w415:errorcluster)
                n365 = local read "LightField Automation out"() -> (w413:refnum<class "LightField Automation.lvclass">)
                n366 = local read "Accumulations"() -> (w412:dbl)
                n367 = property class="Bool (strict)"(reference=w410) -> ("Label.Text"=w411:string)  [unwired: 1 in, 2 out]
                n368 = local read "CCD ROI"() -> (w414:T5)
                n369 = case shown="\"Acquire Spectrum\", Default" w411 {
                  tunnel: [w419 w442 w466 w517] -> w417
                  tunnel: [w420 w441 w465 w516] -> w416
                  tunnel: w415 -> [w424 w443 w467 w516]
                  tunnel: w414 -> [w423 _ _ _]
                  tunnel: w413 -> [w422 w444 w468 w517]
                  tunnel: w412 -> [w421 _ _ _]
                  frame "Acquire Spectrum", Default {
                    n370 = call "Adv_SetROI.vi"("error in (no error)"=w424, "ROI"=w423, "LightField Automation in"=w422) -> ("error out"=w425:errorcluster, "LightField Automation out"=w426:refnum<class "LightField Automation.lvclass">)  [unwired: 7 in]
                    n371 = local read "Acq Mode"() -> (w427:T2)
                    n372 = call "LFA_Capture.vi"("error in (no error)"=w425, "Frames"=w421, "LightField Automation in"=w426) -> ("error out"=w420:errorcluster, "Data"=w418:T1, "LightField Automation out"=w419:refnum<class "LightField Automation.lvclass">)  [unwired: 6 in]
                    "Data" <- w418
                    n373 = case shown="\"Spectrum\", Default" w427 {
                      selector: w427 -> [w432 w437]
                      tunnel: w418 -> [w434 w439]
                      frame "Spectrum", Default {
                        n374 = local read "Wavelength calibration"() -> (w431:dbl[])
                        n375 = Divide(x=1239.841, y=w431) -> (x/y=w429:dbl[])
                        n376 = call "PrepareData4Graph.vi"("Wavelength nm"=w429, "DataLF"=w434, "AcqMode"=w432, "Data type"=T8."Spectre") -> ("Spectrum"=w433:cluster{"Array 2":dbl[], "Array":dbl[]})  [unwired: 4 in, 1 out]
                        n377 = local write "CCD 1D Spectrum Main"(w433) -> ()
                        n378 = property on="Experiment Graph Controls" class="TabCtl (strict)"("Value"=T3."Spectrum Acquisition" ("Experiment Graph Controls")) -> ()  [unwired: 2 in, 2 out]
                      }
                      frame "Image" {
                        n379 = local read "Wavelength calibration"() -> (w438:dbl[])
                        n380 = call "PrepareData4Graph.vi"("Wavelength nm"=w438, "DataLF"=w439, "AcqMode"=w437, "Data type"=T8."Spectre") -> ("Intensity Graph"=w436:dbl[][])  [unwired: 4 in, 1 out]
                        n381 = local write "CCD 2D Image Main"(w436) -> ()
                      }
                    }
                  }
                  frame "Acquire Continuous Spectrum" {
                    n382 = while {
                      tunnel: w444 -> [w452]
                      tunnel: w443 -> [w451]
                      tunnel: [w450] -> w442
                      tunnel: [w449] -> w441
                      stop <- w445 stop-if-true
                      n383 = local read "Accumulations"() -> (w448:dbl)
                      n384 = local read "Acq Mode"() -> (w447:T2)
                      n385 = call "LFA_Capture.vi"("error in (no error)"=w451, "Frames"=w448, "LightField Automation in"=w452) -> ("error out"=w449:errorcluster, "Data"=w446:T1, "LightField Automation out"=w450:refnum<class "LightField Automation.lvclass">)  [unwired: 6 in]
                      n386 = case shown="\"Spectrum\", Default" w447 {
                        selector: w447 -> [w456 w462]
                        tunnel: w446 -> [w458 w464]
                        frame "Spectrum", Default {
                          n387 = local read "Wavelength calibration"() -> (w457:dbl[])
                          n388 = Wait (ms)(milliseconds to wait=u32 150) -> ()  [unwired: 1 out]
                          n389 = call "PrepareData4Graph.vi"("Wavelength nm"=w457, "DataLF"=w458, "AcqMode"=w456, "Data type"=T8."Spectre") -> ("Spectrum"=w454:cluster{"Array 2":dbl[], "Array":dbl[]})  [unwired: 4 in, 1 out]
                          n390 = local write "CCD 1D Spectrum Main"(w454) -> ()
                        }
                        frame "Image" {
                          n391 = local read "Wavelength calibration"() -> (w463:dbl[])
                          n392 = Wait (ms)(milliseconds to wait=u32 150) -> ()  [unwired: 1 out]
                          n393 = call "PrepareData4Graph.vi"("Wavelength nm"=w463, "DataLF"=w464, "AcqMode"=w462, "Data type"=T8."Spectre") -> ("Intensity Graph"=w460:dbl[][])  [unwired: 4 in, 1 out]
                          n394 = local write "CCD 2D Image Main"(w460) -> ()
                        }
                      }
                      n395 = local read "Stop continuous"() -> (w445:bool)
                    }
                  }
                  frame "Acquire Polarisation" {
                    n396 = stacked-sequence {
                      tunnel: w468 -> [_ w496 _]
                      tunnel: w467 -> [_ w495 _]
                      tunnel: [_ w494 _] -> w466
                      tunnel: [_ w493 _] -> w465
                      frame #0 {
                        w481 = TRUE ("Visible")
                        # "shift scale to center"
                        # "from HWP to polarisation units"
                        n397 = property on="Acquire Polarisation" class="Bool (strict)"("Value"=w481) -> ()  [unwired: 2 in, 2 out]
                        n398 = property on="Scan Polarisation Progess Bar" class="Slide (strict)"("Visible"=w481, "Value"=u8 0 ("Scan Polarisation Progess Bar")) -> ()  [unwired: 2 in, 2 out]
                        n399 = property on="CCD 1D Spectrum Main" class="XYGraph (strict)"() -> ("XScale.Maximum"=w473:dbl, "XScale.Minimum"=w472:dbl, "YScale.Minimum"=w471:dbl, "YScale.Maximum"=w470:dbl)  [unwired: 2 in, 2 out]
                        n400 = local read "Polar Start Angle (°)"() -> (w487:dbl)
                        n401 = local read "Polar Step Angle (°)"() -> (w486:dbl)
                        n402 = local read "Scan Polar Params"() -> (w482:refnum<vi>[])
                        n403 = local read "Polar Step Angle (°)"() -> (w478:dbl)
                        n404 = local read "Polar Step Angle (°)"() -> (w475:dbl)
                        n405 = call "Enable&Disable_Controls.vi"("Enum"=enum16{"Enabled", "Disabled", "Disabled&Grayed"}."Disabled&Grayed", "References"=w482) -> ()  [unwired: 1 in]
                        n406 = property on="Polarisation 1D Spectrum" class="XYGraph (strict)"("XScale.Maximum"=w473, "XScale.Minimum"=w472, "YScale.Minimum"=w471, "YScale.Maximum"=w470) -> ()  [unwired: 2 in, 2 out]
                        n407 = Negate(x=w486) -> (-x=w485:dbl)
                        n408 = Multiply(x=2.0, y=w487) -> (x*y=w476:dbl)
                        n409 = property on="Experiment Graph Controls" class="TabCtl (strict)"("Value"=T3."Polarisation Acquisition" ("Experiment Graph Controls")) -> ()  [unwired: 2 in, 2 out]
                        n410 = Subtract(x=w476, y=w475) -> (x-y=w474:dbl)
                        n411 = Multiply(x=2.0, y=w478) -> (x*y=w477:dbl)
                        n412 = Multiply(x=w485, y=0.5) -> ()  [unwired: 1 out]
                        n413 = property on="Polarisation 2D Image" class="IntGraph (strict)"("XScale.Multiplier"=w477, "XScale.Offset"=w474) -> ()  [unwired: 2 in, 2 out]
                      }
                      frame #1 {
                        n414 = local read "Polar mode"() -> (w498:u16)
                        n415 = case shown="3" w498 {
                          tunnel: [w508 w509] -> w499
                          frame 3 {
                            n416 = control-ref of="RotStage Exc Angle (°)"() -> ()  [unwired: 1 out]
                            n417 = control-ref of="RotStage Exc Angle Readout (°)"() -> (w508:refnum<vi>)
                          }
                          frame 2, Default {
                            n418 = control-ref of="RotStage Det Angle (°)"() -> ()  [unwired: 1 out]
                            n419 = control-ref of="RotStage Det Angle Readout (°)"() -> (w509:refnum<vi>)
                          }
                        }
                        n420 = control-ref of="Polarisation 1D Spectrum"() -> (w490:refnum<vi>)
                        n421 = local read "Polar Start Angle (°)"() -> (w507:dbl)
                        n422 = local read "Polar Step Angle (°)"() -> (w505:dbl)
                        n423 = local read "Polar End Angle (°)"() -> (w506:dbl)
                        n424 = local read "ESP 301 COM Port"() -> (w503:refnum<visa-resource-name>)
                        n425 = local read "Acq Time (ms)"() -> (w489:dbl)
                        n426 = control-ref of="Scan Polarisation Progess Bar"() -> (w500:refnum<vi>)
                        n427 = local read "ESP 301 Error"() -> (w504:errorcluster)
                        n428 = local read "Acq Mode"() -> (w497:T2)
                        n429 = control-ref of="Polarisation 2D Image"() -> (w491:refnum<vi>)
                        n430 = call "Polarisation.vi"("VISA resource name"=w503, "Start Angle (°)"=w507, "Exposure time (ms)"=w489, "End Angle (°)"=w506, "ESP301 Error"=w504, "LightField Automation in"=w496, "RotStage Exc Angle Refnum"=w499, "CCD 1D Spectrum Main 3"=w490, "LightField error"=w495, "Acq Mode"=w497, "Step Angle (°)"=w505, "Axis ESP301 / RotStage"=w498, "IntGraph Refnum"=w491, "Slide Refnum"=w500) -> ("Angles"=w492:dbl[], "VISA resource name out"=w501:refnum<visa-resource-name>, "LightField Automation out"=w494:refnum<class "LightField Automation.lvclass">, "LightField error out"=w493:errorcluster, "ESP301 Error out"=w502:errorcluster)  [unwired: 8 in, 1 out]
                        n431 = local write "Angles"(w492) -> ()
                        n432 = local write "ESP 301 COM Port"(w501) -> ()
                        n433 = local write "ESP 301 Error"(w502) -> ()
                      }
                      frame #2 {
                        w513 = FALSE ("Visible")
                        # "set markers to polarisation values"
                        n434 = local read "Angles"() -> (w511:dbl[])
                        n435 = property on="Scan Polarisation Progess Bar" class="Slide (strict)"("Visible"=w513) -> ()  [unwired: 2 in, 2 out]
                        n436 = property on="Acquire Polarisation" class="Bool (strict)"("Value"=w513) -> ()  [unwired: 2 in, 2 out]
                        n437 = local read "Scan Polar Params"() -> (w515:refnum<vi>[])
                        n438 = Multiply(x=2.0, y=w511) -> (x*y=w510:dbl[])
                        n439 = property on="Polarisation 2D Image" class="IntGraph (strict)"("XScale.MarkerVals[]"=w510) -> ()  [unwired: 2 in, 2 out]
                        n440 = call "Enable&Disable_Controls.vi"("Enum"=enum16{"Enabled", "Disabled", "Disabled&Grayed"}."Enabled", "References"=w515) -> ()  [unwired: 1 in]
                      }
                    }
                  }
                  frame "Acquire XY Map" {
                    n441 = disable-structure shown="Disabled" {
                      frame Disabled {
                        n442 = stacked-sequence {
                          frame #0 {
                            n443 = local read "Scan XY Map Params"() -> (w520:refnum<vi>[])
                            n444 = call "Enable&Disable_Controls.vi"("Enum"=enum16{"Enabled", "Disabled", "Disabled&Grayed"}."Disabled&Grayed", "References"=w520) -> ()  [unwired: 1 in]
                            n445 = property on="Experiment Graph Controls" class="TabCtl (strict)"("Value"=T3."XY Intensity Map Acquisition" ("Experiment Graph Controls")) -> ()  [unwired: 2 in, 2 out]
                          }
                          frame #1 {
                            n446 = control-ref of="CCD 1D Spectrum XY Map"() -> (w527:refnum<vi>)
                            n447 = control-ref of="Scan XY Map Progess Bar"() -> (w523:refnum<vi>)
                            n448 = control-ref of="CCD 2D Image XY Map"() -> (w526:refnum<vi>)
                            n449 = control-ref of="Scan X Readout (V)"() -> (w525:refnum<vi>)
                            n450 = control-ref of="Scan Y Readout (V)"() -> (w524:refnum<vi>)
                            n451 = local read "Scan X Tot. Length (V)"() -> (w532:dbl)
                            n452 = local read "Scan Y Tot. Length"() -> (w530:dbl)
                            n453 = control-ref of="Stop XY Map"() -> (w528:refnum<vi>)
                            n454 = local read "Scan X Center (V)"() -> (w534:dbl)
                            n455 = local read "Scan Y Center (V)"() -> (w531:dbl)
                            n456 = local read "Scan X Res. (V)"() -> (w533:dbl)
                            n457 = local read "Scan Y Res. (V)"() -> (w529:dbl)
                            n458 = local read "Scanning Mode"() -> (w535:T7)
                            n459 = local read "Scan Fast Axis"() -> (w521:enum16{"Y", "X"})
                            n460 = Build Array(w528, w527, w526, w523, w525, w524) -> (w522:refnum<vi>[])
                            n461 = call "SubVI_SCAN_FSM300.vi"("X center (Volt)"=w534, "Total Length X (Volt)"=w532, "Scan mode"=w535, "appended array"=w522, "Y center (Volt)"=w531, "Total Length Y (Volt)"=w530, "Resolution X (Volt)"=w533, "Resolution Y (Volt)"=w529, "''fast mooving'' axis"=w521) -> ()  [unwired: 11 in]
                          }
                        }
                      }
                      frame Enabled {
                      }
                    }
                  }
                }
                n462 = local write "LightField Automation error out"(w416) -> ()
                n463 = local write "LightField Automation out"(w417) -> ()
              }
              frame #1 {
                # "AutoSave?"
                n464 = property class="Bool (strict)"(reference=w537) -> ("Label.Text"=w536:string)  [unwired: 1 in, 2 out]
                n465 = local read "Auto< ?"() -> (w538:bool)
                n466 = case shown="True" w538 {
                  tunnel: w536 -> [_ w539]
                  frame False {
                  }
                  frame True {
                    n467 = case shown="\"Acquire Polarisation\"" w539 {
                      frame "Acquire Continuous Spectrum" {
                      }
                      frame "Acquire Polarisation" {
                        n468 = property on="Save Polarisation" class="Bool (strict)"("Val(Sgnl)"=TRUE ("Value (Signaling)")) -> ()  [unwired: 2 in, 2 out]
                      }
                      frame "Acquire XY Map" {
                        n469 = property on="Save XY Map" class="Bool (strict)"("Val(Sgnl)"=TRUE ("Value (Signaling)")) -> ()  [unwired: 2 in, 2 out]
                      }
                      frame "Acquire Spectrum", Default {
                        n470 = property on="Save Spectrum" class="Bool (strict)"("Val(Sgnl)"=TRUE ("Value (Signaling)")) -> ()  [unwired: 2 in, 2 out]
                      }
                    }
                  }
                }
              }
            }
          }
          event "RotStage Exc Angle (°)", "RotStage Det Angle (°)", "Newport Linear Translation Stage Position (mm)": Value Change {
            n471 = event-data() -> ("CtlRef"=w557:refnum<vi>, "NewVal"=w551:dbl)  [unwired: 1 in, 4 out]
            n472 = property class="DigNum (strict)"(reference=w557) -> ("Label.Text"=w555:string)  [unwired: 1 in, 2 out]
            n473 = local read "Excitation Wavelength (nm)"() -> (w547:dbl)
            n474 = local read "Photodiode COM Port"() -> (w549:refnum<visa-resource-name>)
            n475 = local read "Photodiode error out"() -> (w548:errorcluster)
            n476 = local read "ESP 301 COM Port"() -> (w559:refnum<visa-resource-name>)
            n477 = local read "ESP 301 Error"() -> (w558:errorcluster)
            n478 = control-ref of="Excitation Power (uW)"() -> (w550:refnum<vi>)
            n479 = call <instrlib>:"TLPM Set Wavelength.vi"("error in (no error)"=w548, "Wavelength (0.0)"=w547, "instrument handle"=w549) -> ("error out"=w545:errorcluster, "instrument handle out"=w546:refnum<visa-resource-name>)  [unwired: 7 in]
            n480 = case shown="\"RotStage Det Angle (°)\"" w555 {
              tunnel: [2 1 3] -> w556
              tunnel: [w561 w564 w567] -> w552
              tunnel: w551 -> [w560 w563 w566]
              frame "RotStage Det Angle (°)" {
                n481 = local write "RotStage Det Angle (°)"(w560) -> ()
                n482 = control-ref of="RotStage Det Angle Readout (°)"() -> (w561:refnum<vi>)
              }
              frame "Newport Linear Translation Stage Position (mm)" {
                n483 = local write "Newport Linear Translation Stage Position (mm)"(w563) -> ()
                n484 = control-ref of="Newport Linear Translation Stage Position Readout (mm)"() -> (w564:refnum<vi>)
              }
              frame "RotStage Exc Angle (°)", Default {
                n485 = local write "RotStage Exc Angle (°)"(w566) -> ()
                n486 = control-ref of="RotStage Exc Angle Readout (°)"() -> (w567:refnum<vi>)
              }
            }
            n487 = call "Go2Angle.vi"("Excitation Power (uW) 2"=w550, "Position (units)"=w551, "Photodiode error"=w545, "Photodiode"=w546, "ESP301 Error"=w558, "Axis ESP301 / RotStage"=w556, "RotStage Det Angle Readout (°) 4"=w552, "VISA resource name"=w559) -> ("ESP301 Error out"=w553:errorcluster, "Photodiode"=w544:errorcluster, "VISA resource name out"=w554:refnum<visa-resource-name>, "Photodiode out"=w543:refnum<visa-resource-name>)
            n488 = local write "Photodiode COM Port"(w543) -> ()
            n489 = local write "ESP 301 COM Port"(w554) -> ()
            n490 = local write "Photodiode error out"(w544) -> ()
            n491 = local write "ESP 301 Error"(w553) -> ()
          }
          event "RotStage Exc Home", "RotStage Det Home", "Newport Linear Translation Stage Home": Mouse Down {
            n492 = event-data() -> ("CtlRef"=w571:refnum<vi>)  [unwired: 1 in, 7 out]
            n493 = property class="Bool (strict)"(reference=w571) -> ("Label.Text"=w570:string)  [unwired: 1 in, 2 out]
            n494 = case shown="\"Newport Linear Translation Stage Home\"" w570 {
              tunnel: 0.0 -> [w572 w573 w574]
              frame "RotStage Det Home", Default {
                n495 = property on="RotStage Det Angle (°)" class="DigNum (strict)"("Val(Sgnl)"=w572) -> ()  [unwired: 2 in, 2 out]
              }
              frame "Newport Linear Translation Stage Home" {
                n496 = property on="Newport Linear Translation Stage Position (mm)" class="DigNum (strict)"("Val(Sgnl)"=w573) -> ()  [unwired: 2 in, 2 out]
              }
              frame "RotStage Exc Home" {
                n497 = property on="RotStage Exc Angle (°)" class="DigNum (strict)"("Val(Sgnl)"=w574) -> ()  [unwired: 2 in, 2 out]
              }
            }
          }
          event "RotStage Exc Jog Backward", "RotStage Det Jog Backward", "RotStage Exc Jog Forward", "RotStage Det Jog Forward", "Newport Linear Translation Stage Jog Forward", "Newport Linear Translation Stage Jog Backward": Mouse Down {
            n498 = event-data() -> ("CtlRef"=w576:refnum<vi>)  [unwired: 1 in, 7 out]
            n499 = property class="Bool (strict)"(reference=w576) -> ("Label.Text"=w575:string)  [unwired: 1 in, 2 out]
            n500 = case shown="\"Newport Linear Translation Stage Jog Backward\"" w575 {
              frame "RotStage Det Jog Backward" {
                n501 = local read "RotStage Det Angle Readout (°)"() -> (w579:dbl)
                n502 = local read "RotStage Det Angle Step (°)"() -> (w578:dbl)
                n503 = Subtract(x=w579, y=w578) -> (x-y=w577:dbl)
                n504 = property on="RotStage Det Angle (°)" class="DigNum (strict)"("Val(Sgnl)"=w577) -> ()  [unwired: 2 in, 2 out]
              }
              frame Default {
              }
              frame "RotStage Det Jog Forward" {
                n505 = local read "RotStage Det Angle Readout (°)"() -> (w581:dbl)
                n506 = local read "RotStage Det Angle Step (°)"() -> (w582:dbl)
                n507 = Add(x=w581, y=w582) -> (x+y=w580:dbl)
                n508 = property on="RotStage Det Angle (°)" class="DigNum (strict)"("Val(Sgnl)"=w580) -> ()  [unwired: 2 in, 2 out]
              }
              frame "RotStage Exc Jog Forward" {
                n509 = local read "RotStage Exc Angle Readout (°)"() -> (w585:dbl)
                n510 = local read "RotStage Exc Angle Step (°)"() -> (w584:dbl)
                n511 = Add(x=w585, y=w584) -> (x+y=w583:dbl)
                n512 = property on="RotStage Exc Angle (°)" class="DigNum (strict)"("Val(Sgnl)"=w583) -> ()  [unwired: 2 in, 2 out]
              }
              frame "Newport Linear Translation Stage Jog Forward" {
                n513 = local read "Newport Linear Translation Stage Position Readout (mm)"() -> (w588:dbl)
                n514 = local read "Newport Linear Translation Stage Step (mm)"() -> (w587:dbl)
                n515 = Add(x=w588, y=w587) -> (x+y=w586:dbl)
                n516 = property on="Newport Linear Translation Stage Position (mm)" class="DigNum (strict)"("Val(Sgnl)"=w586) -> ()  [unwired: 2 in, 2 out]
              }
              frame "Newport Linear Translation Stage Jog Backward" {
                n517 = local read "Newport Linear Translation Stage Position Readout (mm)"() -> (w591:dbl)
                n518 = local read "Newport Linear Translation Stage Step (mm)"() -> (w590:dbl)
                n519 = Subtract(x=w591, y=w590) -> (x-y=w589:dbl)
                n520 = property on="Newport Linear Translation Stage Position (mm)" class="DigNum (strict)"("Val(Sgnl)"=w589) -> ()  [unwired: 2 in, 2 out]
              }
              frame "RotStage Exc Jog Backward" {
                n521 = local read "RotStage Exc Angle Readout (°)"() -> (w594:dbl)
                n522 = local read "RotStage Exc Angle Step (°)"() -> (w593:dbl)
                n523 = Subtract(x=w594, y=w593) -> (x-y=w592:dbl)
                n524 = property on="RotStage Exc Angle (°)" class="DigNum (strict)"("Val(Sgnl)"=w592) -> ()  [unwired: 2 in, 2 out]
              }
            }
          }
          event "RotStage Exc Velocity (°/s)", "RotStage Det Velocity (°/s)", "Newport Linear Translation Stage Velocity (mm/s)": Value Change {
            n525 = event-data() -> ("CtlRef"=w601:refnum<vi>, "NewVal"=w599:dbl)  [unwired: 1 in, 4 out]
            n526 = property class="DigNum (strict)"(reference=w601) -> ("Label.Text"=w600:string)  [unwired: 1 in, 2 out]
            n527 = local read "ESP 301 COM Port"() -> (w598:refnum<visa-resource-name>)
            n528 = local read "ESP 301 Error"() -> (w597:errorcluster)
            n529 = case shown="\"RotStage Det Velocity (°/s)\"" w600 {
              tunnel: w599 -> [w605 _ w610 w620]
              tunnel: w598 -> [w606 w609 w612 w619]
              tunnel: w597 -> [w607 w608 w613 w618]
              tunnel: [w603 w609 w615 w617] -> w596
              tunnel: [w602 w608 w614 w616] -> w595
              frame "Newport Linear Translation Stage Velocity (mm/s)" {
                n530 = call "Set Velocity.vi"("error in (no error)"=w607, "Velocity (units/s)"=w605, "Axis (1)"=1, "VISA resource name"=w606) -> ("error out"=w602:errorcluster, "VISA resource name out"=w603:refnum<visa-resource-name>)  [unwired: 2 in]
              }
              frame Default {
              }
              frame "RotStage Det Velocity (°/s)" {
                n531 = call "Set Velocity.vi"("error in (no error)"=w613, "Velocity (units/s)"=w610, "Axis (1)"=2, "VISA resource name"=w612) -> ("error out"=w614:errorcluster, "VISA resource name out"=w615:refnum<visa-resource-name>)  [unwired: 2 in]
              }
              frame "RotStage Exc Velocity (°/s)" {
                n532 = call "Set Velocity.vi"("error in (no error)"=w618, "Velocity (units/s)"=w620, "Axis (1)"=3, "VISA resource name"=w619) -> ("error out"=w616:errorcluster, "VISA resource name out"=w617:refnum<visa-resource-name>)  [unwired: 2 in]
              }
            }
            n533 = local write "ESP 301 COM Port"(w596) -> ()
            n534 = local write "ESP 301 Error"(w595) -> ()
          }
          event "Exposure Time (ms)": Value Change {
            n535 = event-data() -> ("NewVal"=w622:dbl)  [unwired: 1 in, 5 out]
            n536 = local write "Acq Time (ms)"(w622) -> ()
            n537 = local read "LightField Automation error out"() -> (w631:errorcluster)
            n538 = local read "LightField Automation out"() -> (w630:refnum<class "LightField Automation.lvclass">)
            n539 = Divide(x=w622, y=1000.0) -> (x/y=w623:dbl)
            n540 = call "Exp_CCD_GetExposureTime.vi"("error in (no error)"=w631, "LightField Automation in"=w630) -> ("error out"=w624:errorcluster, "Exposure Time (s)"=w629:dbl, "LightField Automation out"=w625:refnum<class "LightField Automation.lvclass">)  [unwired: 7 in]
            n541 = Equal?(x=w629, y=w623) -> (x = y?=w628:bool)
            n542 = case shown="False" w628 {
              tunnel: [w638 w654] -> w627
              tunnel: [w637 w655] -> w626
              tunnel: w625 -> [w635 w655]
              tunnel: w624 -> [w634 w654]
              tunnel: w623 -> [w636 _]
              tunnel: w622 -> [w633 _]
              frame False {
                n543 = stacked-sequence {
                  seq-local: [w643 _] -> [_ w653]
                  seq-local: [w642 _] -> [_ w652]
                  tunnel: w636 -> [w641 _]
                  tunnel: w635 -> [w640 _]
                  tunnel: w634 -> [w639 _]
                  tunnel: [_ w653] -> w638
                  tunnel: [_ w652] -> w637
                  tunnel: w633 -> [_ w649]
                  frame #0 {
                    n544 = call "Exp_CCD_SetExposureTime.vi"("error in (no error)"=w639, "Exposure Time (s)"=w641, "LightField Automation in"=w640) -> ("error out"=w643:errorcluster, "LightField Automation out"=w642:refnum<class "LightField Automation.lvclass">)  [unwired: 7 in]
                  }
                  frame #1 {
                    n545 = Format Into String(format string="%5d", initial string="Exposure time set to ", w649) -> (resulting string=w645:string)  [unwired: 1 in, 1 out]
                    n546 = local read "Log file"() -> (w651:string)
                    n547 = Concatenate Strings(w645, " ms") -> (w644:string)
                    n548 = call "Write2LogFile.vi"("Add to log file"=w644, "Log file before"=w651) -> ("Log file after"=w650:string)
                    n549 = local write "Log file"(w650) -> ()
                  }
                }
              }
              frame True {
              }
            }
            n550 = local write "LightField Automation out"(w626) -> ()
            n551 = local write "LightField Automation error out"(w627) -> ()
          }
          event "Acq Time (ms)": Value Change {
            n552 = event-data() -> ("NewVal"=w656:dbl)  [unwired: 1 in, 5 out]
            n553 = local read "Acq Mode"() -> (w657:T2)
            n554 = case shown="\"Image\"" w657 {
              tunnel: w656 -> [w658 w659]
              frame "Image" {
                n555 = property on="Exposure Time (ms)" class="DigNum (strict)"("Val(Sgnl)"=w658) -> ()  [unwired: 2 in, 2 out]
              }
              frame "Spectrum", Default {
                n556 = property on="Exposure Time (ms)" class="DigNum (strict)"("Val(Sgnl)"=w659) -> ()  [unwired: 2 in, 2 out]
              }
            }
          }
          event "ThorCam Init": Mouse Down {
            n557 = event-data() -> ()  [unwired: 1 in, 8 out]
            n558 = local read "ThorCam Init"() -> (w661:bool)
            n559 = local read "ThorCam Reference"() -> (w662:refnum<k24>)
            n560 = local read "ThorCam Visu"() -> (w663:refnum<k24>)
            n561 = local read "Thorcam Error"() -> (w664:errorcluster)
            n562 = case shown="True" w661 {
              tunnel: w664 -> [_ w695]
              tunnel: w663 -> [_ w692]
              tunnel: w662 -> [w675 w689]
              tunnel: [w665 w676] -> w660
              frame False {
                n563 = property class="Camera"(reference=w675) -> (error out=w673:errorcluster, "Acquisition"=w674:refnum<k24>)  [unwired: 1 in, 1 out]
                n564 = invoke class="Acquisition" method="Stop"(reference=w674, error in=w673) -> (reference out=w672:refnum<k24>, error out=w671:errorcluster, "Stop"=w666:i32)  [unwired: 1 in]
                n565 = invoke class="Acquisition" method="ToString"(reference=w672, error in=w671) -> (reference out=w670:refnum<k24>, error out=w669:errorcluster, "ToString"=w668:string)  [unwired: 1 in]
                n566 = Close Reference(reference=w670, error in (no error)=w669) -> (error out=w667:errorcluster)
                n567 = call "uc480_Error_Handling.vi"("Error Code"=w666, "Error String"=w668, "Error In"=w667) -> ("Error Out"=w665:errorcluster)  [unwired: 8 in]
              }
              frame True {
                n568 = call "uc480_SubVI_Example_StartLive.vi"("Error"=w695, ".NET (Reference)"=w689) -> ("Error"=w691:errorcluster)  [unwired: 9 in]
                n569 = property class="PictureBox"(reference=w692, error in=w691, "Width"=640, "Height"=512) -> (error out=w690:errorcluster, "Handle"=w681:refnum<k24>)  [unwired: 1 out]
                n570 = property class="Camera"(reference=w689, error in=w690) -> (reference out=w685:refnum<k24>, error out=w688:errorcluster, "Memory"=w687:refnum<k24>)
                n571 = invoke class="Memory" method="GetActive"(reference=w687, error in=w688) -> (reference out=w677:refnum<k24>, error out=w686:errorcluster, "s32MemId"=w682:i32)  [unwired: 2 in, 1 out]
                n572 = property class="Camera"(reference=w685, error in=w686) -> (error out=w683:errorcluster, "Display"=w684:refnum<k24>)  [unwired: 1 out]
                n573 = invoke class="Display" method="Render"(reference=w684, error in=w683, "memID"=w682, "windowHandle"=w681) -> (reference out=w680:refnum<k24>, error out=w679:errorcluster)  [unwired: 1 in, 3 out]
                n574 = Close Reference(reference=w680, error in (no error)=w679) -> (error out=w678:errorcluster)
                n575 = Close Reference(reference=w677, error in (no error)=w678) -> (error out=w676:errorcluster)
              }
            }
            n576 = local write "Thorcam Error"(w660) -> ()
          }
          event "CCD 1D Spectrum Main": Cursor Release {
            n577 = event-data() -> ()  [unwired: 1 in, 9 out]
            n578 = stacked-sequence {
              seq-local: [w697 _] -> [_ w705]
              seq-local: [w696 _] -> [_ w704]
              frame #0 {
                n579 = property on="CCD 1D Spectrum Main" class="XYGraph (strict)"("Active Cursor"=u32 0, "Active Cursor"=u32 1) -> ("Cursor.Cursor X"=w697:dbl, "Cursor.Cursor X"=w696:dbl)  [unwired: 2 in, 2 out]
                n580 = local write "CCD 1D Spectrum Main Cursor"(w697) -> ()
                n581 = local write "CCD 1D Spectrum Main Cursor 2"(w696) -> ()
              }
              frame #1 {
                n582 = call "Cursors2Freq.vi"("Cursor 1 eV"=w705, "Cursor 2 eV"=w704) -> ("Cursor dE"=w703:dbl, "Cursor 1 nm"=w702:dbl, "Cursor 2 nm"=w701:dbl, "Cursor dnm"=w700:dbl)
                n583 = local write "CCD 1D Spectrum Main deltaE"(w703) -> ()
                n584 = local write "CCD 1D Spectrum Main Cursor 1 nm"(w702) -> ()
                n585 = local write "CCD 1D Spectrum Main Cursor 2 nm"(w701) -> ()
                n586 = Multiply(x=w700, y=1e-09) -> (x*y=w706:dbl)
                n587 = local write "CCD 1D Spectrum Main deltanm"(w706) -> ()
              }
            }
          }
          event "Shutter Ctrls", "KCubeSolenoidControl": Mouse Down {
            # "1 open"
            n588 = event-data() -> ()  [unwired: 1 in, 8 out]
            n589 = local read "KCube Shutter Device Reference"() -> (w710:refnum<k24>)
            n590 = control-ref of="Shutter Ctrls"() -> (w714:refnum<vi>)
            n591 = property on="Property Node" class="Ring (strict)"(reference=w714) -> (reference out=w717:refnum<vi>, "NumItems"=w718:u32)  [unwired: 1 in, 1 out]
            n592 = invoke class="KCubeSolenoid" method="GetOperatingState"(reference=w710) -> ("GetOperatingState"=w708:i32)  [unwired: 2 in, 2 out]
            n593 = property on="Property Node" class="Ring (strict)"(reference=w717) -> ("Value"=w716:u16)  [unwired: 1 in, 2 out]
            n594 = Equal?(x=w708, y=2.0) -> (x = y?=w713:bool)
            n595 = Equal?(x=w716, y=u16 0) -> (x = y?=w712:bool)
            n596 = Or(x=w713, y=w712) -> (x .or. y?=w711:bool)
            n597 = case shown="True" w711 {
              frame True {
                n598 = local read "KCube Shutter Device Reference"() -> (w720:refnum<k24>)
                n599 = invoke class="KCubeSolenoid" method="SetOperatingState"(reference=w720, "eState"=1) -> ()  [unwired: 2 in, 4 out]
              }
              frame False {
                n600 = local read "KCube Shutter Device Reference"() -> (w722:refnum<k24>)
                n601 = invoke class="KCubeSolenoid" method="SetOperatingState"(reference=w722, "eState"=2) -> ()  [unwired: 2 in, 4 out]
              }
            }
            n602 = case shown="False" w711 {
              tunnel: w718 -> [w723 w736]
              tunnel: w717 -> [w724 w735]
              frame False {
                n603 = for {
                  N: w723 -> [w727]
                  tunnel: w724 -> [w725]
                  i -> [w726]
                  n604 = flat-sequence {
                    tunnel: w726 -> [w730]
                    tunnel: w727 -> [w733]
                    tunnel: w725 -> [w728]
                    frame #0 {
                      n605 = Add(x=w730, y=1) -> (x+y=w731:i32)
                      n606 = Subtract(x=w733, y=w731) -> (x-y=w732:i32)
                      n607 = property on="Property Node" class="Ring (strict)"(reference=w728, "Value"=w732) -> ()  [unwired: 1 in, 2 out]
                    }
                    frame #1 {
                      n608 = Wait (ms)(milliseconds to wait=u32 70) -> ()  [unwired: 1 out]
                    }
                  }
                }
              }
              frame True {
                n609 = for {
                  N: w736 -> [_]
                  tunnel: w735 -> [w737]
                  i -> [w738]
                  n610 = flat-sequence {
                    tunnel: w738 -> [w739]
                    tunnel: w737 -> [w740]
                    frame #0 {
                      n611 = property on="Property Node" class="Ring (strict)"(reference=w740, "Value"=w739) -> ()  [unwired: 1 in, 2 out]
                    }
                    frame #1 {
                      n612 = Wait (ms)(milliseconds to wait=u32 70) -> ()  [unwired: 1 out]
                    }
                  }
                }
              }
            }
          }
          event "TEC Output", "TEC Temperature", "Laser on? Control": Mouse Down; "Laser Diode Current Set": Value Change {
            n613 = event-data() -> ("CtlRef"=w746:refnum<vi>)  [unwired: 1 in, 3 out]
            n614 = local read "Photodiode COM Port"() -> (w745:refnum<visa-resource-name>)
            n615 = local read "Photodiode error out"() -> (w744:errorcluster)
            n616 = local read "Diode Driver COM"() -> (w751:refnum<visa-resource-name>)
            n617 = local read "Diode Driver Error"() -> (w750:errorcluster)
            n618 = property class="Ctl"(reference=w746) -> ("Label.Text"=w747:string)  [unwired: 1 in, 2 out]
            n619 = case shown="\"Laser Diode Current Set\"" w747 {
              tunnel: w751 -> [w757 w768 w795 w829]
              tunnel: w750 -> [w756 w767 w794 w828]
              tunnel: [w755 w765 w793 w823] -> w749
              tunnel: [w754 w766 w792 w822] -> w748
              tunnel: w745 -> [w752 w760 w789 w819]
              tunnel: w744 -> [w753 w759 w788 w820]
              tunnel: [w752 w762 w787 w819] -> w743
              tunnel: [w753 w761 w786 w820] -> w742
              frame "TEC Temperature" {
                n620 = call <instrlib>:"TL4000 Measure Temperature.vi"("error in (no error)"=w756, "instrument handle"=w757) -> ("error out"=w754:errorcluster, "Temperature"=w758:dbl, "instrument handle out"=w755:refnum<visa-resource-name>)  [unwired: 7 in]
                n621 = local write "TEC Temperature"(w758) -> ()
              }
              frame "Laser on? Control" {
                n622 = flat-sequence {
                  tunnel: w768 -> [w776]
                  tunnel: w767 -> [w775]
                  tunnel: [w774] -> w764
                  tunnel: [w773] -> w763
                  tunnel: [w784] -> w765
                  tunnel: [w785] -> w766
                  tunnel: w764 -> [w785]
                  tunnel: w763 -> [w784]
                  tunnel: [w783] -> w762
                  tunnel: [w782] -> w761
                  tunnel: w760 -> [w781]
                  tunnel: w759 -> [w780]
                  frame #0 {
                    n623 = call <instrlib>:"TL4000 Get LD Output State.vi"("error in (no error)"=w775, "instrument handle"=w776) -> ("error out"=w770:errorcluster, "LD Output"=w772:bool, "instrument handle out"=w771:refnum<visa-resource-name>)  [unwired: 7 in]
                    n624 = case shown="True" w772 {
                      selector: w772 -> [w777 w778]
                      frame False {
                        n625 = property on="TEC Output" class="Bool (strict)"("Visible"=w777) -> ()  [unwired: 2 in, 2 out]
                      }
                      frame True {
                        n626 = property on="TEC Output" class="Bool (strict)"("Visible"=w778) -> ()  [unwired: 2 in, 2 out]
                      }
                    }
                    n627 = Not(x=w772) -> (.not. x?=w769:bool)
                    n628 = property on="Laser Safety" class="Ring (strict)"("Visible"=w769) -> ()  [unwired: 2 in, 2 out]
                    n629 = local write "Laser on?"(w769) -> ()
                    n630 = call <instrlib>:"TL4000 Switch LD Output.vi"("error in (no error)"=w770, "LD Output (Off)"=w769, "instrument handle"=w771) -> ("error out"=w774:errorcluster, "instrument handle out"=w773:refnum<visa-resource-name>)  [unwired: 7 in]
                  }
                  frame #1 {
                    n631 = call <instrlib>:"TLPM Measure Power.vi"("error in (no error)"=w780, "instrument handle"=w781) -> ("error out"=w782:errorcluster, "Power"=w779:dbl, "instrument handle out"=w783:refnum<visa-resource-name>)  [unwired: 7 in]
                    n632 = local write "Excitation Power (uW)"(w779) -> ()
                  }
                }
              }
              frame "Laser Diode Current Set" {
                n633 = flat-sequence {
                  tunnel: w795 -> [w804]
                  tunnel: w794 -> [w803]
                  tunnel: [w799] -> w791
                  tunnel: [w798] -> w790
                  tunnel: [w817] -> w792
                  tunnel: [w818] -> w793
                  tunnel: w791 -> [w818]
                  tunnel: w790 -> [w817]
                  tunnel: w789 -> [w816]
                  tunnel: w788 -> [w815]
                  tunnel: [w814] -> w787
                  tunnel: [w813] -> w786
                  frame #0 {
                    n634 = local read "Laser Diode Current Set"() -> (w796:dbl)
                    n635 = call <instrlib>:"TL4000 Get Laser Diode Current Setpoint.vi"("error in (no error)"=w803, "instrument handle"=w804) -> ("error out"=w800:errorcluster, "Laser Diode Current Setpoint"=w802:dbl, "instrument handle out"=w801:refnum<visa-resource-name>)  [unwired: 7 in]
                    n636 = Not Equal?(x=w796, y=w802) -> (x != y?=w797:bool)
                    n637 = case shown="True" w797 {
                      tunnel: w801 -> [w806 w811]
                      tunnel: w800 -> [w805 w810]
                      tunnel: [w806 w809] -> w799
                      tunnel: [w805 w808] -> w798
                      tunnel: w796 -> [_ w807]
                      frame False {
                      }
                      frame True {
                        n638 = call <instrlib>:"TL4000 Set Laser Diode Current Setpoint.vi"("error in (no error)"=w810, "Laser Diode Current Setpoint (0.0)"=w807, "instrument handle"=w811) -> ("error out"=w808:errorcluster, "instrument handle out"=w809:refnum<visa-resource-name>)  [unwired: 7 in]
                      }
                    }
                  }
                  frame #1 {
                    n639 = call <instrlib>:"TLPM Measure Power.vi"("error in (no error)"=w815, "instrument handle"=w816) -> ("error out"=w813:errorcluster, "Power"=w812:dbl, "instrument handle out"=w814:refnum<visa-resource-name>)  [unwired: 7 in]
                    n640 = local write "Excitation Power (uW)"(w812) -> ()
                  }
                }
              }
              frame "TEC Output", Default {
                n641 = call <instrlib>:"TL4000 Get TEC Output State.vi"("error in (no error)"=w828, "instrument handle"=w829) -> ("error out"=w826:errorcluster, "TEC Output"=w830:bool, "instrument handle out"=w827:refnum<visa-resource-name>)  [unwired: 7 in]
                n642 = Not(x=w830) -> (.not. x?=w821:bool)
                n643 = local write "TEC Output"(w821) -> ()
                n644 = property on="Laser on? Control" class="Bool (strict)"("Visible"=w821) -> ()  [unwired: 2 in, 2 out]
                n645 = call <instrlib>:"TL4000 Switch TEC Output.vi"("error in (no error)"=w826, "TEC Output (Off)"=w821, "instrument handle"=w827) -> ("error out"=w824:errorcluster, "instrument handle out"=w825:refnum<visa-resource-name>)  [unwired: 7 in]
                n646 = case shown="True" w821 {
                  tunnel: w825 -> [w832 w839]
                  tunnel: w824 -> [w831 w838]
                  tunnel: [w832 w835] -> w823
                  tunnel: [w831 w834] -> w822
                  frame False {
                  }
                  frame True {
                    n647 = while {
                      tunnel: w839 -> [w853]
                      tunnel: w838 -> [w852]
                      tunnel: [w846] -> w837
                      tunnel: [w845] -> w836
                      stop <- w840 stop-if-true
                      n648 = call <instrlib>:"TL4000 Measure Temperature.vi"("error in (no error)"=w852, "instrument handle"=w853) -> ("error out"=w846:errorcluster, "Temperature"=w843:dbl, "instrument handle out"=w845:refnum<visa-resource-name>)  [unwired: 7 in]
                      n649 = Wait (ms)(milliseconds to wait=u32 50) -> ()  [unwired: 1 out]
                      n650 = local write "TEC Temperature"(w843) -> ()
                      n651 = Subtract(x=w843, y=25.0) -> (x-y=w850:dbl)
                      n652 = Absolute Value(x=w850) -> (abs(x)=w849:dbl)
                      n653 = Less?(x=w849, y=0.01) -> (x < y?=w844:bool)
                      n654 = Equal?(x=w843, y=0.0) -> (x = y?=w841:bool)
                      n655 = Or(x=w844, y=w841) -> (x .or. y?=w840:bool)
                    }
                    n656 = call <instrlib>:"TL4000 Measure Temperature.vi"("error in (no error)"=w837, "instrument handle"=w836) -> ("error out"=w834:errorcluster, "Temperature"=w833:dbl, "instrument handle out"=w835:refnum<visa-resource-name>)  [unwired: 7 in]
                    n657 = local write "TEC Temperature"(w833) -> ()
                  }
                }
              }
            }
            n658 = local write "Diode Driver COM"(w749) -> ()
            n659 = local write "Diode Driver Error"(w748) -> ()
            n660 = local write "Photodiode COM Port"(w743) -> ()
            n661 = local write "Photodiode error out"(w742) -> ()
          }
          event "Center Wavelength (nm)": Value Change {
            n662 = event-data() -> ("NewVal"=w854:dbl)  [unwired: 1 in, 5 out]
            n663 = local read "LightField Automation error out"() -> (w861:errorcluster)
            n664 = local read "LightField Automation out"() -> (w862:refnum<class "LightField Automation.lvclass">)
            n665 = call "spec_GetCenterWavelength.vi"("error in (no error)"=w861, "LightField Automation in"=w862) -> ("error out"=w857:errorcluster, "Center Wavelength"=w860:dbl, "LightField Automation out"=w858:refnum<class "LightField Automation.lvclass">)  [unwired: 7 in]
            n666 = Equal?(x=w854, y=w860) -> (x = y?=w859:bool)
            n667 = case shown="False" w859 {
              tunnel: w858 -> [w867 w887]
              tunnel: w857 -> [w866 w886]
              tunnel: [w863 w887] -> w856
              tunnel: [w864 w886] -> w855
              tunnel: w854 -> [w865 _]
              frame False {
                n668 = stacked-sequence {
                  seq-local: [w871 _] -> [_ w885]
                  seq-local: [w870 _] -> [_ w884]
                  seq-local: [w868 _] -> [_ w883]
                  tunnel: w867 -> [w875 _]
                  tunnel: w866 -> [w874 _]
                  tunnel: w865 -> [w868 _]
                  tunnel: [_ w885] -> w864
                  tunnel: [_ w884] -> w863
                  frame #0 {
                    n669 = call "spec_SetCenterWavelength.vi"("error in (no error)"=w874, "Center Wavelength"=w868, "LightField Automation in"=w875) -> ("error out"=w872:errorcluster, "LightField Automation out"=w873:refnum<class "LightField Automation.lvclass">)  [unwired: 7 in]
                    n670 = call "spec_getCalibration.vi"("error in (no error)"=w872, "LightField Automation in"=w873) -> ("error out"=w871:errorcluster, "ColumnCalibration"=w869:dbl[], "LightField Automation out"=w870:refnum<class "LightField Automation.lvclass">)  [unwired: 7 in]
                    n671 = local write "Wavelength calibration"(w869) -> ()
                  }
                  frame #1 {
                    n672 = Format Into String(format string="%3.2f", initial string="Wavelength set to ", w883) -> (resulting string=w881:string)  [unwired: 1 in, 1 out]
                    n673 = local read "Log file"() -> (w878:string)
                    n674 = Concatenate Strings(w881, " nm") -> (w879:string)
                    n675 = call "Write2LogFile.vi"("Add to log file"=w879, "Log file before"=w878) -> ("Log file after"=w877:string)
                    n676 = local write "Log file"(w877) -> ()
                  }
                }
              }
              frame True {
              }
            }
            n677 = local write "LightField Automation out"(w856) -> ()
            n678 = local write "LightField Automation error out"(w855) -> ()
          }
          event "CCD 1D Spectrum Main  Cursor2WL 1 Mono 1", "CCD 1D Spectrum Main  Cursor2WL 2 Mono 1": Mouse Down {
            n679 = event-data() -> ("CtlRef"=w889:refnum<vi>)  [unwired: 1 in, 7 out]
            n680 = property class="Bool (strict)"(reference=w889) -> ("Label.Text"=w888:string)  [unwired: 1 in, 2 out]
            n681 = case shown="\"CCD 1D Spectrum Main  Cursor2WL 2\"" w888 {
              tunnel: [w891 w892] -> w890
              frame "CCD 1D Spectrum Main  Cursor2WL 1", Default {
                n682 = local read "CCD 1D Spectrum Main Cursor 1 nm"() -> (w891:dbl)
              }
              frame "CCD 1D Spectrum Main  Cursor2WL 2" {
                n683 = local read "CCD 1D Spectrum Main Cursor 2 nm"() -> (w892:dbl)
              }
            }
            n684 = property on="Center Wavelength (nm)" class="DigNum (strict)"("Val(Sgnl)"=w890) -> ()  [unwired: 2 in, 2 out]
          }
          event "Cryostat": Value Change {
            n685 = event-data() -> ("NewVal"=w893:enum16{"Montana", "Oxford"})  [unwired: 1 in, 5 out]
            n686 = case shown="\"Oxford\"" w893 {
              frame "Oxford" {
                w894 = FALSE
                n687 = property on="FSM Up" class="Bool (strict)"("Visible"=w894) -> ()  [unwired: 2 in, 2 out]
                n688 = property on="FSM Left" class="Bool (strict)"("Visible"=w894) -> ()  [unwired: 2 in, 2 out]
                n689 = property on="FSM Axis Step" class="DigNum (strict)"("Visible"=w894) -> ()  [unwired: 2 in, 2 out]
                n690 = property on="FSM Down" class="Bool (strict)"("Visible"=w894) -> ()  [unwired: 2 in, 2 out]
                n691 = property on="FSM Right" class="Bool (strict)"("Visible"=w894) -> ()  [unwired: 2 in, 2 out]
              }
              frame "Montana" {
                w895 = TRUE
                n692 = property on="FSM Up" class="Bool (strict)"("Visible"=w895) -> ()  [unwired: 2 in, 2 out]
                n693 = property on="FSM Left" class="Bool (strict)"("Visible"=w895) -> ()  [unwired: 2 in, 2 out]
                n694 = property on="FSM Axis Step" class="DigNum (strict)"("Visible"=w895) -> ()  [unwired: 2 in, 2 out]
                n695 = property on="FSM Down" class="Bool (strict)"("Visible"=w895) -> ()  [unwired: 2 in, 2 out]
                n696 = property on="FSM Right" class="Bool (strict)"("Visible"=w895) -> ()  [unwired: 2 in, 2 out]
              }
            }
          }
          event "Shutter Mode": Value Change {
            # "1 Active == Laser on / Shutter off\n2 Inactive == Laser off / Shutter on\n\nThere are 4 operating modes for shutter:\n1 Manual\n2 Single Toggle\n3 Automatic Toggle\n4 Triggered"
            n697 = event-data() -> ()  [unwired: 1 in, 6 out]
            n698 = local read "KCube Shutter Device Reference"() -> (w897:refnum<k24>)
            n699 = local read "Shutter Mode"() -> (w896:i32)
            n700 = invoke class="KCubeSolenoid" method="SetOperatingMode"(reference=w897, "mode"=w896) -> ()  [unwired: 2 in, 4 out]
          }
          event "Save Spectrum", "Save Spectrum N", "Save XY Map", "Save Polarisation": Value Change {
            n701 = event-data() -> ("CtlRef"=w899:refnum<vi>)  [unwired: 1 in, 3 out]
            n702 = property class="Bool (strict)"(reference=w899) -> ("Label.Text"=w898:string)  [unwired: 1 in, 2 out]
            n703 = stacked-sequence {
              tunnel: w898 -> [w900 _]
              frame #0 {
                n704 = Wait (ms)(milliseconds to wait=u32 500) -> ()  [unwired: 1 out]
                n705 = local read "Center Wavelength (nm)"() -> (w906:dbl)
                n706 = local read "Excitation Power (uW)"() -> (w910:dbl)
                n707 = local read "Exposure Time (ms)"() -> (w907:dbl)
                n708 = local read "Experiment Name"() -> (w905:string)
                n709 = local read "Temperature (K)"() -> (w909:dbl)
                n710 = local read "Excitation Source"() -> (w908:enum16{"P", "CW"})
                n711 = local read "Comment"() -> (w904:string)
                n712 = local read "Log file"() -> (w902:string)
                n713 = case shown="\"Save Spectrum\", Default" w900 {
                  tunnel: w910 -> [_ _ _ w923]
                  tunnel: w909 -> [_ _ _ w922]
                  tunnel: w908 -> [_ _ _ w921]
                  tunnel: w907 -> [_ _ _ w920]
                  tunnel: w906 -> [_ _ _ w919]
                  tunnel: w905 -> [_ _ _ w918]
                  tunnel: w904 -> [_ _ _ w917]
                  tunnel: w902 -> [w911 w912 w913 w916]
                  tunnel: [w911 w912 w913 w915] -> w901
                  frame "Save Spectrum N" {
                  }
                  frame "Save XY Map" {
                  }
                  frame "Save Polarisation" {
                  }
                  frame "Save Spectrum", Default {
                    n714 = local read "Acq Mode"() -> (w914:T2)
                    n715 = case shown="\"Spectrum\", Default" w914 {
                      tunnel: w923 -> [w937 w950]
                      tunnel: w922 -> [w936 w949]
                      tunnel: w921 -> [w935 w948]
                      tunnel: w920 -> [w934 w947]
                      tunnel: w919 -> [w933 w946]
                      tunnel: w918 -> [w932 w945]
                      tunnel: w917 -> [w931 w944]
                      tunnel: w916 -> [w930 w943]
                      tunnel: [w929 w942] -> w915
                      tunnel: w914 -> [w924 w940]
                      frame "Spectrum", Default {
                        n716 = local read "CCD 1D Spectrum Main"() -> (w927:cluster{dbl[], dbl[]})
                        n717 = Unbundle(w927) -> (w926:dbl[], w925:dbl[])
                        n718 = call "Format&SaveDataWithAttributes.vi"("Comment"=w931, "Exp_Temperature_K"=w936, "Det_Mono1_CenterWL_nm"=w933, "Exc_ExcitationPower_uW"=w937, "Exc_ExcitationSource"=w935, "Det_AcqTime_ms"=w934, "Measurement type"=T9."Spectrum", "Data_PLInt_cts"=w925, "FileName"=w932, "Data_Wavelength_nm"=w926, "Acq Mode"=w924, "Log File In"=w930) -> ("Log File Out"=w929:string)  [unwired: 14 in, 1 out]
                      }
                      frame "Image" {
                        n719 = local read "Wavelength calibration"() -> (w939:dbl[])
                        n720 = local read "CCD 2D Image Main"() -> (w938:dbl[][])
                        n721 = call "Format&SaveDataWithAttributes.vi"("Comment"=w944, "Exp_Temperature_K"=w949, "Det_Mono1_CenterWL_nm"=w946, "Exc_ExcitationPower_uW"=w950, "Exc_ExcitationSource"=w948, "Det_AcqTime_ms"=w947, "Measurement type"=T9."Spectrum", "FileName"=w945, "Data_Wavelength_nm"=w939, "Acq Mode"=w940, "Log File In"=w943, "Data_CCD_px"=w938) -> ("Log File Out"=w942:string)  [unwired: 14 in, 1 out]
                      }
                    }
                  }
                }
                n722 = local write "Log file"(w901) -> ()
              }
              frame #1 {
                w951 = FALSE
                n723 = local write "Save XY Map"(w951) -> ()
                n724 = local write "Save Polarisation"(w951) -> ()
                n725 = local write "Save Spectrum N"(w951) -> ()
                n726 = local write "Save Spectrum"(w951) -> ()
              }
            }
          }
          event "Auto< ?": Value Change {
            n727 = event-data() -> ("NewVal"=w952:bool)  [unwired: 1 in, 5 out]
            n728 = case shown="True" w952 {
              frame False {
                w953 = TRUE ("Visible")
                n729 = property on="Save Spectrum N" class="Bool (strict)"("Visible"=w953) -> ()  [unwired: 2 in, 2 out]
                n730 = property on="Save XY Map" class="Bool (strict)"("Visible"=w953) -> ()  [unwired: 2 in, 2 out]
                n731 = property on="Save Spectrum" class="Bool (strict)"("Visible"=w953) -> ()  [unwired: 2 in, 2 out]
                n732 = property on="Save Polarisation" class="Bool (strict)"("Visible"=w953) -> ()  [unwired: 2 in, 2 out]
              }
              frame True {
                w954 = FALSE ("Visible")
                n733 = property on="Save Spectrum N" class="Bool (strict)"("Visible"=w954) -> ()  [unwired: 2 in, 2 out]
                n734 = property on="Save XY Map" class="Bool (strict)"("Visible"=w954) -> ()  [unwired: 2 in, 2 out]
                n735 = property on="Save Spectrum" class="Bool (strict)"("Visible"=w954) -> ()  [unwired: 2 in, 2 out]
                n736 = property on="Save Polarisation" class="Bool (strict)"("Visible"=w954) -> ()  [unwired: 2 in, 2 out]
              }
            }
          }
        }
      }
    }
    frame #2 {
      # "Shutdown: close all open references and connections"
      n737 = stacked-sequence {
        frame #0 {
          # "Shutdown all connections"
          n738 = local read "Initialise all devices?"() -> (w955:bool)
          n739 = case shown="True" w955 {
            frame False {
              # "No devices to deactivate"
            }
            frame True {
              # "Deactivate all the selected devices"
              n740 = stacked-sequence {
                frame #0 {
                  # "Message to user"
                  n741 = local read "Log file"() -> (w958:string)
                  n742 = call "Write2LogFile.vi"("Add to log file"="Closing all connections ...", "Log file before"=w958) -> ("Log file after"=w957:string)
                  n743 = local write "Log file"(w957) -> ()
                }
                frame #1 {
                  # "KCubes: 1 Shutter + 3 Piezos"
                  n744 = local read "KCubes Piezo On?"() -> (w960:bool)
                  n745 = case shown="True" w960 {
                    frame False {
                    }
                    frame True {
                      # "Close piezo controls and shutter device"
                      n746 = local read "KCubePiezoControl Y Reference"() -> (w963:refnum<k24>)
                      n747 = local read "KCubePiezoControl X Reference"() -> (w962:refnum<k24>)
                      n748 = local read "KCubePiezoControl Z Reference"() -> (w964:refnum<k24>)
                      n749 = invoke class="KCubePiezoControl" method="CloseDevice"(reference=w963) -> ()  [unwired: 2 in, 3 out]
                      n750 = invoke class="KCubePiezoControl" method="CloseDevice"(reference=w962) -> ()  [unwired: 2 in, 3 out]
                      n751 = invoke class="KCubePiezoControl" method="CloseDevice"(reference=w964) -> ()  [unwired: 2 in, 3 out]
                    }
                  }
                  n752 = local read "KCube Shutter On?"() -> (w959:bool)
                  n753 = case shown="True" w959 {
                    frame False {
                    }
                    frame True {
                      n754 = local read "KCubeSolenoidControl Reference"() -> (w961:refnum<k24>)
                      n755 = invoke class="KCubeSolenoidControl" method="CloseDevice"(reference=w961) -> ()  [unwired: 2 in, 3 out]
                    }
                  }
                }
                frame #2 {
                  # "LightField: SpectraPro Mono + CCD"
                  n756 = local read "LightField On?"() -> (w965:bool)
                  n757 = case shown="True" w965 {
                    frame False {
                    }
                    frame True {
                      n758 = local read "LightField Automation error out"() -> (w966:errorcluster)
                      n759 = local read "LightField Automation out"() -> (w967:refnum<class "LightField Automation.lvclass">)
                      n760 = call "LFA_Close.vi"("error in (no error)"=w966, "LightField Automation in"=w967) -> ()  [unwired: 8 in, 2 out]
                    }
                  }
                }
                frame #3 {
                  # "ESP 301: 2 rotation stages + 1 linear translation stage"
                  n761 = local read "ESP 301 On?"() -> (w968:bool)
                  n762 = case shown="True" w968 {
                    frame False {
                    }
                    frame True {
                      n763 = local read "ESP 301 COM Port"() -> (w970:refnum<visa-resource-name>)
                      n764 = local read "ESP 301 Error"() -> (w969:errorcluster)
                      n765 = call "Close.vi"("error in (no error)"=w969, "VISA resource name"=w970) -> ()  [unwired: 9 in, 1 out]
                    }
                  }
                }
                frame #4 {
                  # "ESP 300: Mono Jobin Yvon"
                  n766 = local read "ESP 300 On?"() -> (w971:bool)
                  n767 = case shown="True" w971 {
                    frame False {
                    }
                    frame True {
                      n768 = local read "ESP 300 COM Port"() -> (w972:refnum<visa-resource-name>)
                      n769 = local read "ESP300 Error"() -> (w973:errorcluster)
                      n770 = call "Uninit Communication.vi"("error in (no error)"=w973, "VISA resource name in"=w972) -> ()  [unwired: 9 in, 1 out]
                    }
                  }
                }
                frame #5 {
                  # "turn off laser output, TEC and close connection"
                  # "448.3nm Laser Diode + Temp Controller & Driver"
                  n771 = local read "Laser Comm On?"() -> (w974:bool)
                  n772 = case shown="True" w974 {
                    frame False {
                    }
                    frame True {
                      w975 = FALSE ("LD Output (Off)")
                      n773 = local read "Diode Driver COM"() -> (w982:refnum<visa-resource-name>)
                      n774 = local read "Diode Driver Error"() -> (w981:errorcluster)
                      n775 = Not(x=w975) -> (.not. x?=w976:bool)
                      n776 = call <instrlib>:"TL4000 Switch LD Output.vi"("error in (no error)"=w981, "LD Output (Off)"=w975, "instrument handle"=w982) -> ("error out"=w980:errorcluster, "instrument handle out"=w979:refnum<visa-resource-name>)  [unwired: 7 in]
                      n777 = property on="Laser Safety" class="Ring (strict)"("Visible"=w975) -> ()  [unwired: 2 in, 2 out]
                      n778 = local write "Laser on? Control"(w975) -> ()
                      n779 = local write "Laser on?"(w975) -> ()
                      n780 = property on="TEC Output" class="Bool (strict)"("Visible"=w976) -> ()  [unwired: 2 in, 2 out]
                      n781 = call <instrlib>:"TL4000 Switch TEC Output.vi"("error in (no error)"=w980, "TEC Output (Off)"=w975, "instrument handle"=w979) -> ("error out"=w977:errorcluster, "instrument handle out"=w978:refnum<visa-resource-name>)  [unwired: 7 in]
                      n782 = call <instrlib>:"TL4000 Close.vi"("error in (no error)"=w977, "instrument handle"=w978) -> ("error out"=w983:errorcluster)  [unwired: 9 in]
                      n783 = local write "Diode Driver Error"(w983) -> ()
                      n784 = local write "TEC Output"(w975) -> ()
                    }
                  }
                }
                frame #6 {
                  # "Thorlabs USB photodiode"
                  n785 = local read "PM16-120 On?"() -> (w984:bool)
                  n786 = case shown="True" w984 {
                    frame False {
                    }
                    frame True {
                      n787 = local read "Photodiode handle out"() -> (w989:refnum<visa-resource-name>)
                      n788 = local read "Photodiode error out"() -> (w988:errorcluster)
                      n789 = call <instrlib>:"TLPM Measure Power.vi"("error in (no error)"=w988, "instrument handle"=w989) -> ("error out"=w986:errorcluster, "Power"=w985:dbl, "instrument handle out"=w987:refnum<visa-resource-name>)  [unwired: 7 in]
                      n790 = call <instrlib>:"TLPM Close.vi"("error in (no error)"=w986, "instrument handle"=w987) -> ("error out"=w990:errorcluster)  [unwired: 9 in]
                      n791 = local write "Excitation Power (uW)"(w985) -> ()
                      n792 = local write "Photodiode error out"(w990) -> ()
                    }
                  }
                }
              }
            }
          }
        }
        frame #1 {
          # "Save log file & empty strings for next operation"
          n793 = stacked-sequence {
            frame #0 {
              # "save log file"
              n794 = local read "Experiment Name"() -> (w993:string)
              n795 = local read "Log file"() -> (w994:string)
              n796 = call "CreatePath.vi"("filetype"=enum16{".h5", ".txt"}.".txt", "FileName"=w993) -> ("File path"=w991:path)
              n797 = Write to Text File(file (use dialog)=w991, text=w994) -> ()  [unwired: 2 in, 3 out]
            }
            frame #1 {
              w995 = ""
              # "reset log file and \ncomment to empty"
              n798 = local write "Log file"(w995) -> ()
              n799 = local write "Comment"(w995) -> ()
            }
          }
        }
      }
    }
  }
  n800 = control-ref of="Polar Start Angle (°)"() -> (w1:refnum<vi>)
  n801 = disable-structure shown="Enabled" {
    frame Disabled {
    }
    frame Enabled {
      # "XYZ objective piezos and shutter"
      # "connected through"
      # "XY Scanning measurements"
      # "Polarisation measurement"
      # "Graphs"
      # "Spectrum with CCD"
      # "Spectrum with APDs"
      # "Acquire controls"
      # "Save controls"
      # "CCD"
      # "MonochromatorS"
      # "Rotation stages PR50PP"
      # "Main"
      # "Photodiode PM16-120"
      # "Steering mirror FSM 300"
      # "Settings for instrumentation"
      # "Contrôle manip GH013"
      n802 = property on="CCD 1D Spectrum Main Energy Scale" class="XYGraph (strict)"("Plot.Visible?"=FALSE ("Plot.Visible"), "Plot.Line Width"=u8 0) -> ()  [unwired: 2 in, 2 out]
      n803 = local write "Photodiode Status"(FALSE) -> ()
      n804 = property on="Polarisation 1D Spectrum Energy Scale" class="XYGraph (strict)"("Plot.Visible?"=FALSE ("Plot.Visible"), "Plot.Line Width"=u8 0) -> ()  [unwired: 2 in, 2 out]
      n805 = control-ref of="Scan Fast Axis"() -> (w1004:refnum<vi>)
      n806 = control-ref of="Scan X Num. Pts"() -> (w1000:refnum<vi>)
      n807 = control-ref of="Scanning Mode"() -> (w1003:refnum<vi>)
      n808 = control-ref of="Scan Y Center (V)"() -> (w999:refnum<vi>)
      n809 = control-ref of="Scan X Center (V)"() -> (w1002:refnum<vi>)
      n810 = control-ref of="Scan Y Res. (V)"() -> (w998:refnum<vi>)
      n811 = control-ref of="Scan Y Num. Pts"() -> (w997:refnum<vi>)
      n812 = control-ref of="Scan X Res. (V)"() -> (w1001:refnum<vi>)
      n813 = Build Array(w1004, w1003, w1002, w1001, w1000, w999, w998, w997) -> (→"Scan XY Map Params":refnum<vi>[])
    }
  }
  n814 = control-ref of="Polar Step Angle (°)"() -> (w3:refnum<vi>)
  n815 = control-ref of="Polar End Angle (°)"() -> (w2:refnum<vi>)
  n816 = control-ref of="Polar mode"() -> (w4:refnum<vi>)
  n817 = Build Array(w4, w1, w2, w3) -> (→"Scan Polar Params":refnum<vi>[])
